vi "Main_HSI.vi"() -> ()   [LabVIEW 2018]
uses:
  <vilib>/vision/Image Controls.llb/IMAQ Image.ctl
  Hyperspectral_Analysis_v2018 - Copie/HSI.llb/Commande 1.ctl
panel:
  out "SPECTRUM ON ROI":cluster{"WAVELENGTH":dbl[], "SPECTRUM":dbl[]}[](graph)
  out "IMAGE U8":u8[][][](array[numeric])
  in  "BAND TO VISUALIZE 3":i32=45 caption="BAND TO VISUALIZE"
  in  "BAND TO VISUALIZE 2":i32=45 caption="BAND TO VISUALIZE"
  in  "GREEN BAND 3":i32=45 caption="GREEN BAND"
  in  "BLUE BAND 3":i32=45 caption="BLUE BAND"
  in  "RED BAND 3":i32=45 caption="RED BAND"
  in  "GREEN BAND 2":i32=45 caption="GREEN BAND"
  in  "BLUE BAND 2":i32=45 caption="BLUE BAND"
  in  "RED BAND 2":i32=45 caption="RED BAND"
  out "path 2":path
  out "path":path
  out "VISU RGB IMAGE":T1
  in  "GREEN BAND":i32=45
  in  "BLUE BAND":i32=45
  in  "RED BAND":i32=45
  out "DISPLAY RGB IMAGE":T1(plugin-control)
  in  "START SPECTRA CALCULATION":bool
  in  "BACK TO MAIN 3":bool
  in  "BACK TO MAIN 2":bool
  in  "IMAGES FOLDER":path
  out "SPECTRA OF CLUSTER CENTERS":cluster{"WAVELENGTH":dbl[], "SPECTRUM":dbl[]}[](graph)
  in  "XSTART":i16=1
  in  "# Clusters":i16=4
  in  "YEND":i16=300
  in  "XEND":i16=300
  in  "YSTART":i16=1
  in  "# Iterations":i16=100
  out "ANALYSIS IN PROGRESS":u16(slide) max=100 step=10 scale=0.0..100.0 scale format="%.1f"
  out "CLUSTER":T1(plugin-control)
  in  "CALCULATE CLUSTER":bool
  out "ROI":T2
  in  "IMAGE PATH":path
  out "CURRENT PICTURE ANALYZED":string
  in  "NEXT IMAGE":bool
  out "WAVELENGTH":sgl[](array[numeric])=[470.0, 472.8859, 475.7718, 478.6577, 481.5436, 484.4295, 487.3154, 490.2013, 493.0872, 495.9732, 498.8591, 501.745, 504.6309, 507.5168, 510.4027, 513.2886, 516.1745, 519.0604, 521.9463, 524.8322, 527.7181, 530.604, 533.4899, 536.3758, 539.2617, 542.1477, 545.0336, 547.9195, 550.8054, 553.6913, 556.5772, 559.4631, 562.349, 565.2349, 568.1208, 571.0067, 573.8926, 576.7785, 579.6644, 582.5503, 585.4362, 588.3221, 591.2081, 594.094, 596.9799, 599.8658, 602.7517, 605.6376, 608.5235, 611.4094, 614.2953, 617.1812, 620.0671, 622.953, 625.8389, 628.7248, 631.6107, 634.4966, 637.3826, 640.2685, 643.1544, 646.0403, 648.9262, 651.8121, 654.698, 657.5839, 660.4698, 663.3557, 666.2416, 669.1275, 672.0134, 674.8993, 677.7852, 680.6711, 683.557, 686.443, 689.3289, 692.2148, 695.1007, 697.9866, 700.8725, 703.7584, 706.6443, 709.5302, 712.4161, 715.302, 718.1879, 721.0738, 723.9597, 726.8456, 729.7315, 732.6174, 735.5034, 738.3893, 741.2752, 744.1611, 747.047, 749.9329, 752.8188, 755.7047, 758.5906, 761.4765, 764.3624, 767.2483, 770.1342, 773.0201, 775.906, 778.7919, 781.6779, 784.5638, 787.4497, 790.3356, 793.2215, 796.1074, 798.9933, 801.8792, 804.7651, 807.651, 810.5369, 813.4228, 816.3087, 819.1946, 822.0805, 824.9664, 827.8523, 830.7383, 833.6242, 836.5101, 839.396, 842.2819, 845.1678, 848.0537, 850.9396, 853.8255, 856.7114, 859.5973, 862.4832, 865.3691, 868.255, 871.1409, 874.0268, 876.9128, 879.7987, 882.6846, 885.5705, 888.4564, 891.3423, 894.2282, 897.1141, 900.0]
  out "CUBE":sgl[][][](array[numeric])
  in  "BACK TO MAIN":bool
  out "VISU 1 LAYER U8":T1
  in  "BAND TO VISUALIZE":i32=45
  in  "WAVELENGTH NUMBER":i32=150
  in  "IMAGES FOLDER PATH":path
  in  "START CLUSTERIZATION":bool
  out "DISPLAY 1 BAND":T1(plugin-control)
  in  "QUIT":bool=TRUE
  in  "ROI AUTO":bool=TRUE
  in  "DEMO":bool=TRUE
  in  "AVERAGE SPECTRUM":bool=TRUE
  in  "CLUSTERIZATION":bool
  # "Hyperspectral Analysis v1.0"
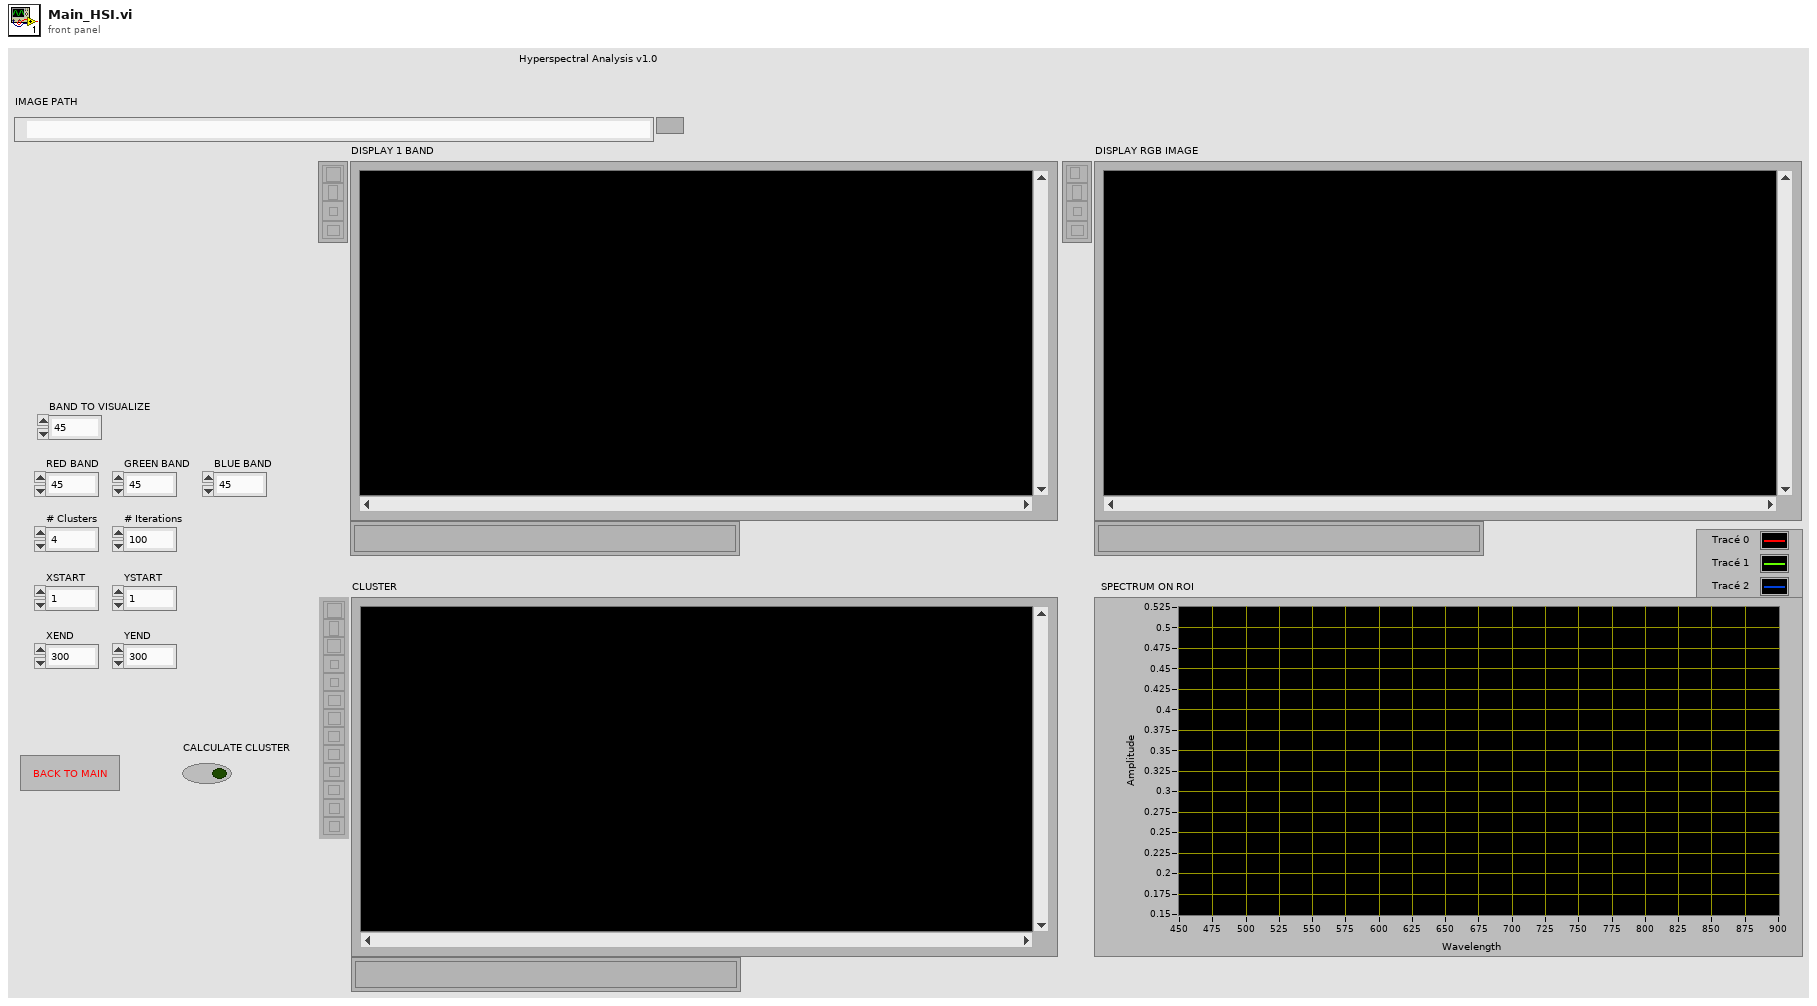
[diagram p1: front panel]
types:
  T1 = typedef "IMAQ Image.ctl" = refnum<image>
  T2 = cluster{"Global Rectangle":i32[], "Contours":cluster{"Contour Type":u32, "ROI Type":u32, "Points":i32[]}[]}
  T3 = enum8{"Enabled", "Disabled", "Disabled and Grayed Out"}
  T4 = typedef "Commande 1.ctl" = cluster{"Tableau":dbl[], "Tableau 2":dbl[]}[]
  T5 = typedef "Image Type" = u32
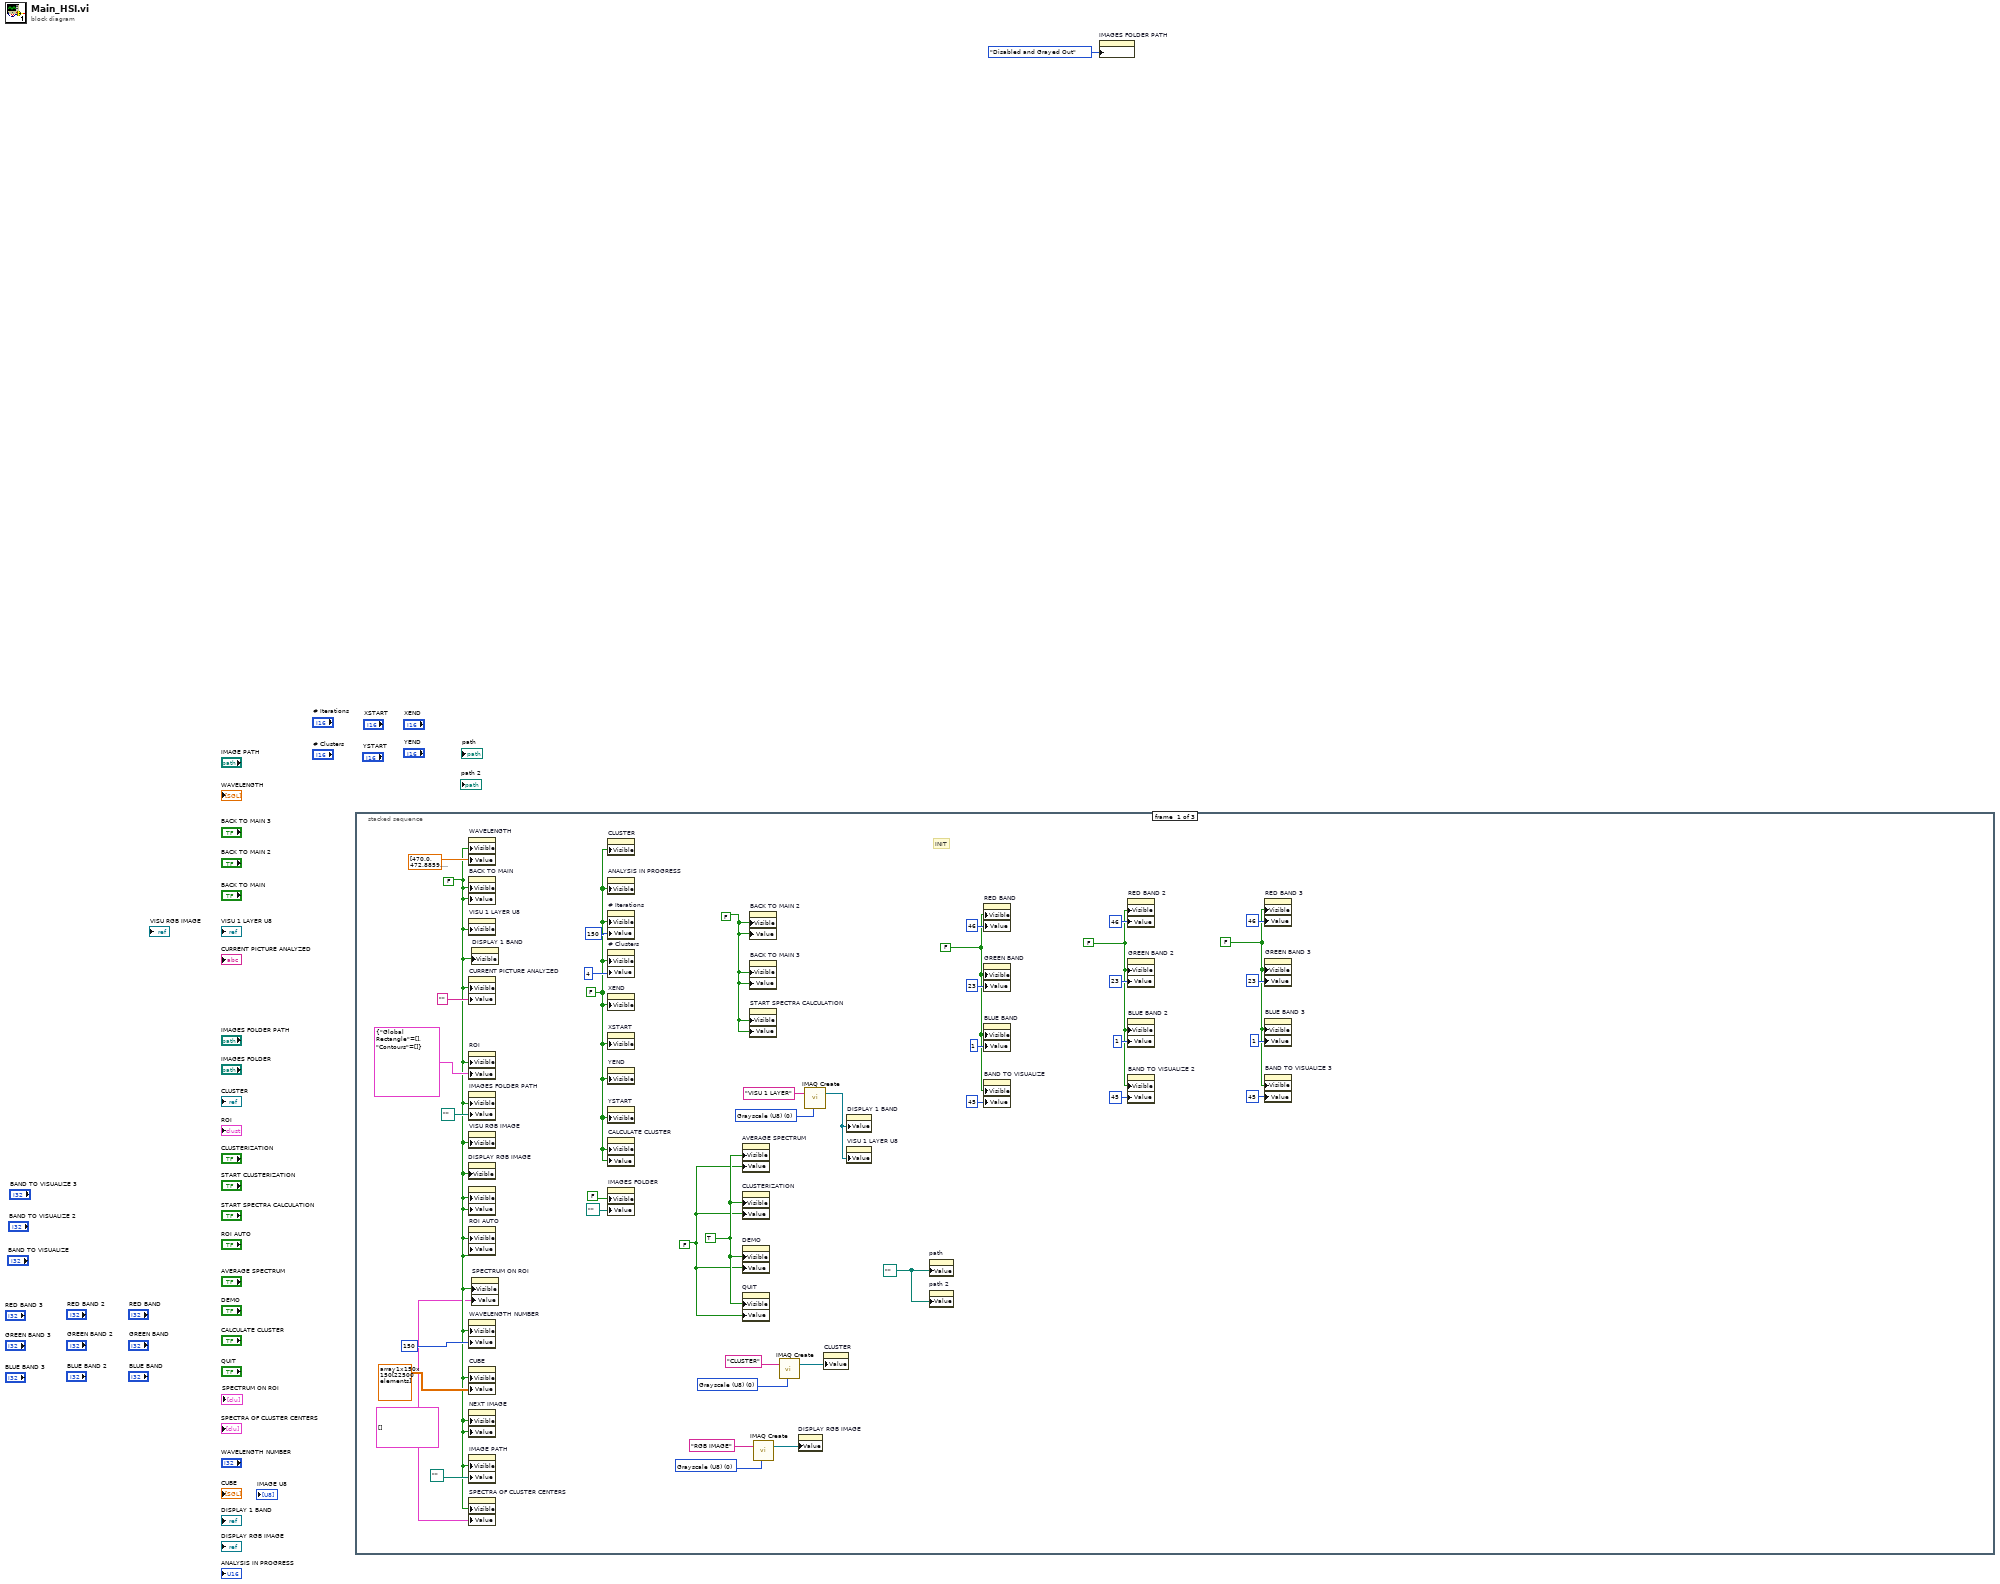
[diagram p0: block diagram]
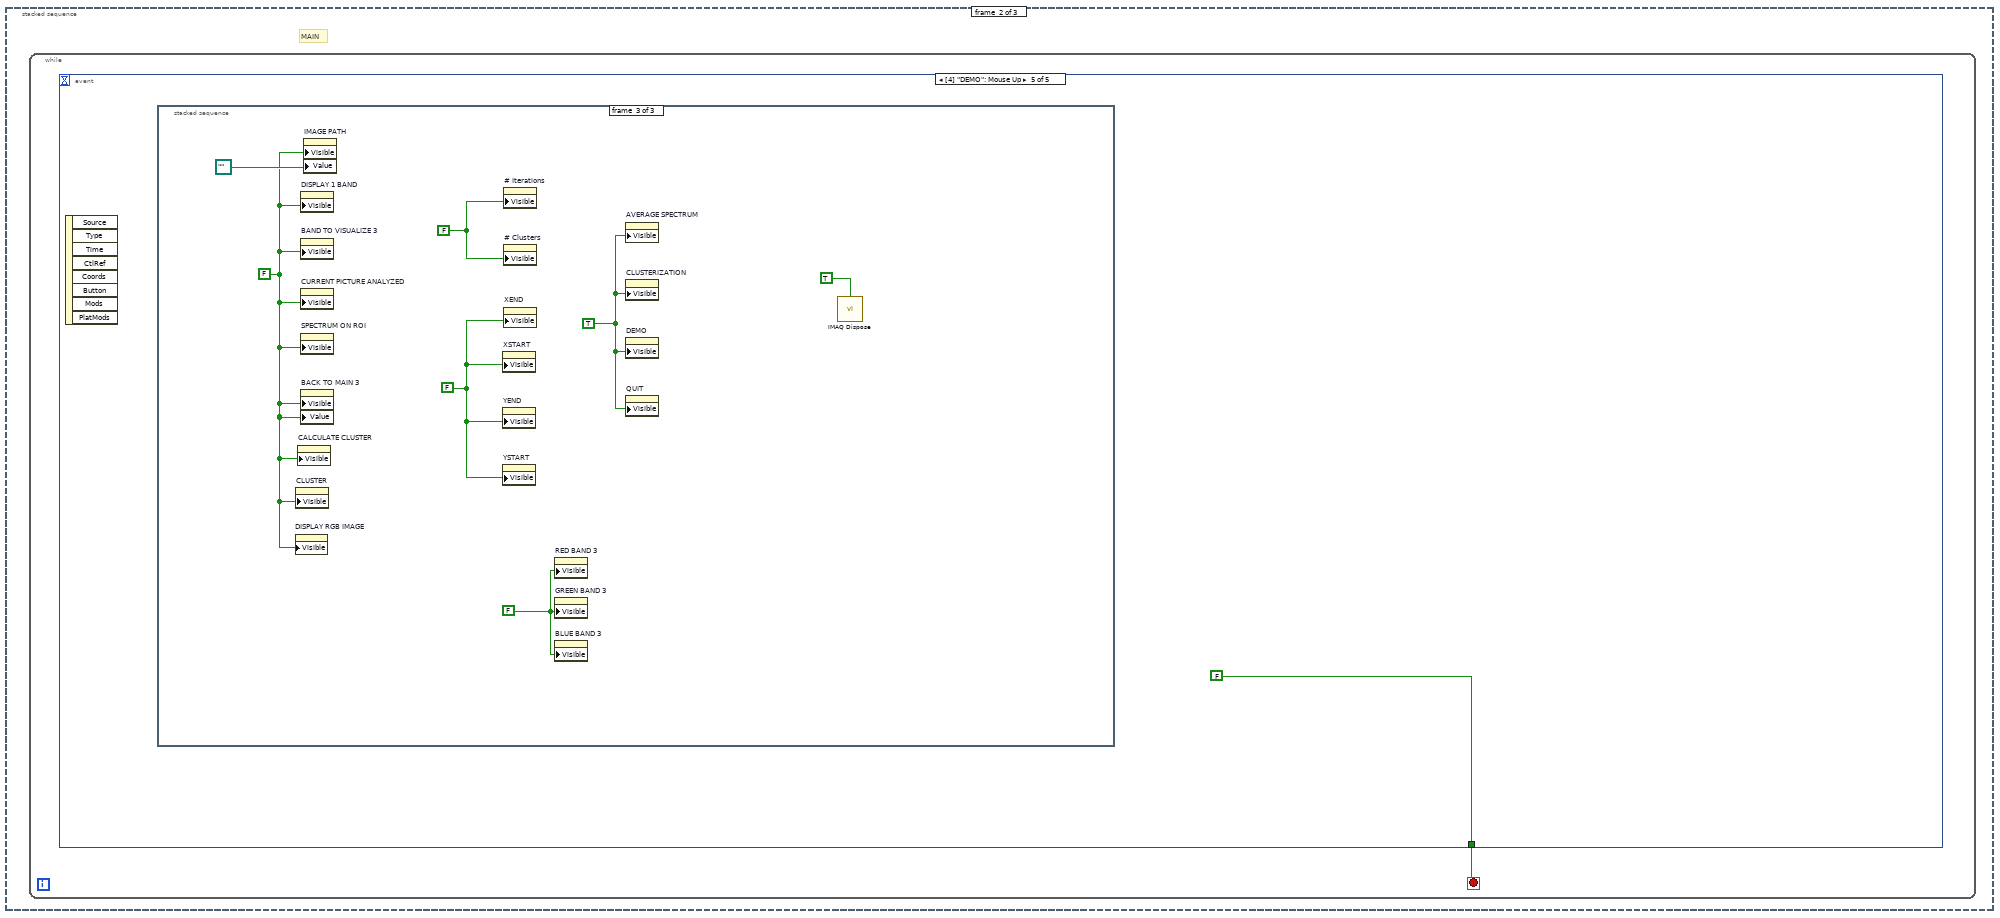
[diagram p2: hidden frame]
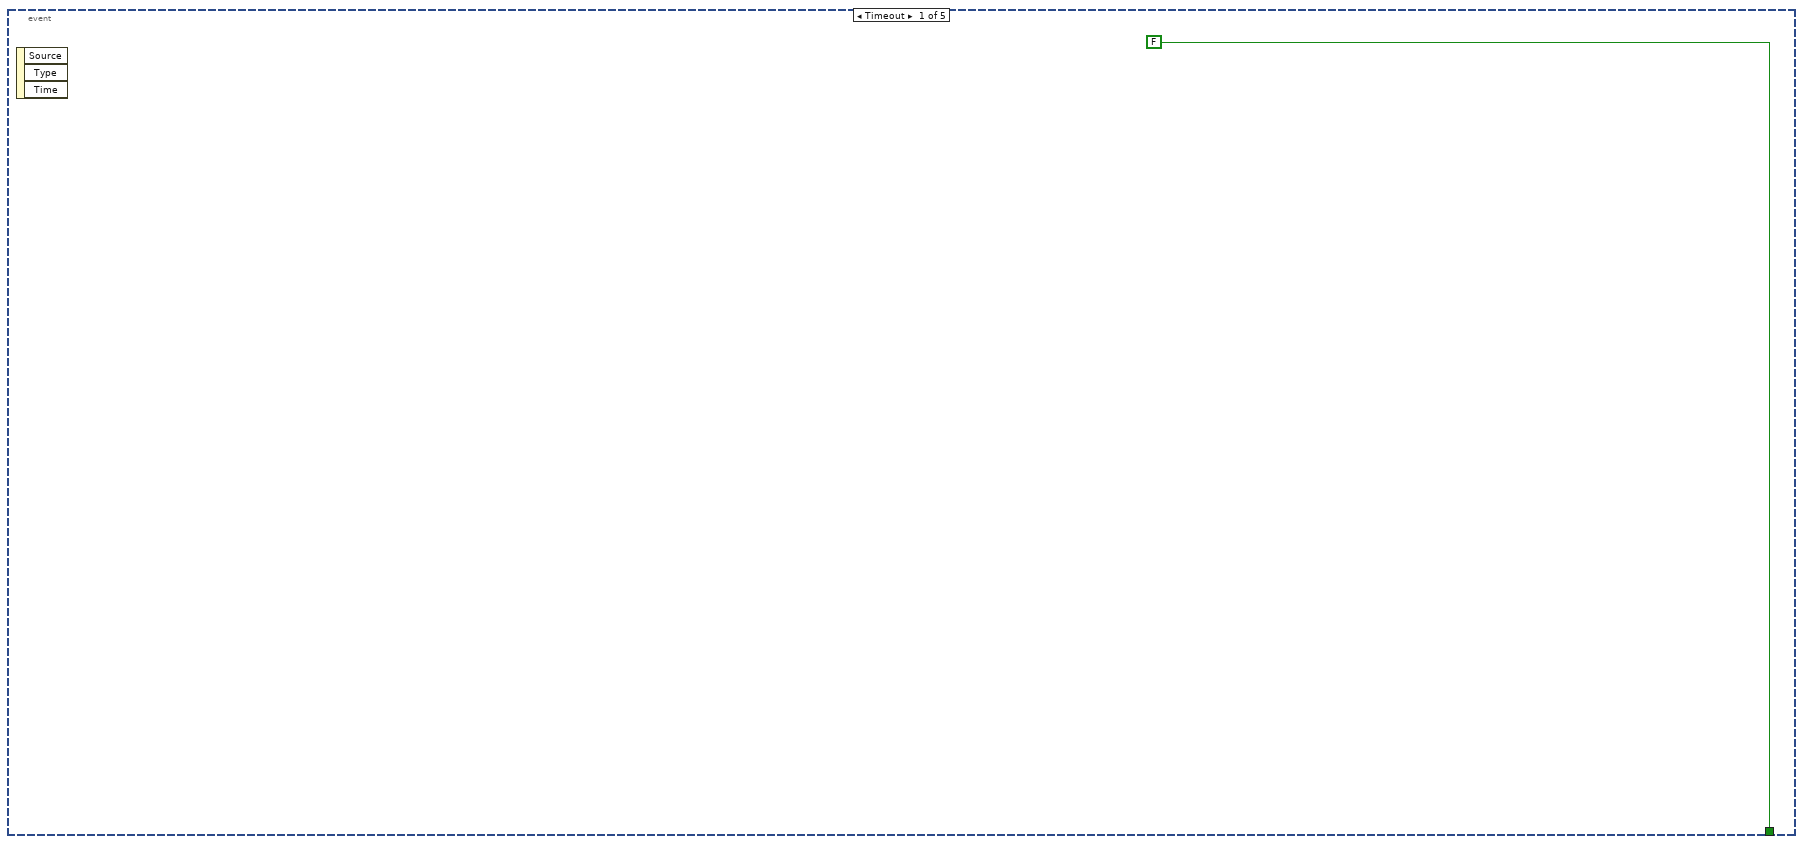
[diagram p3: hidden frame]
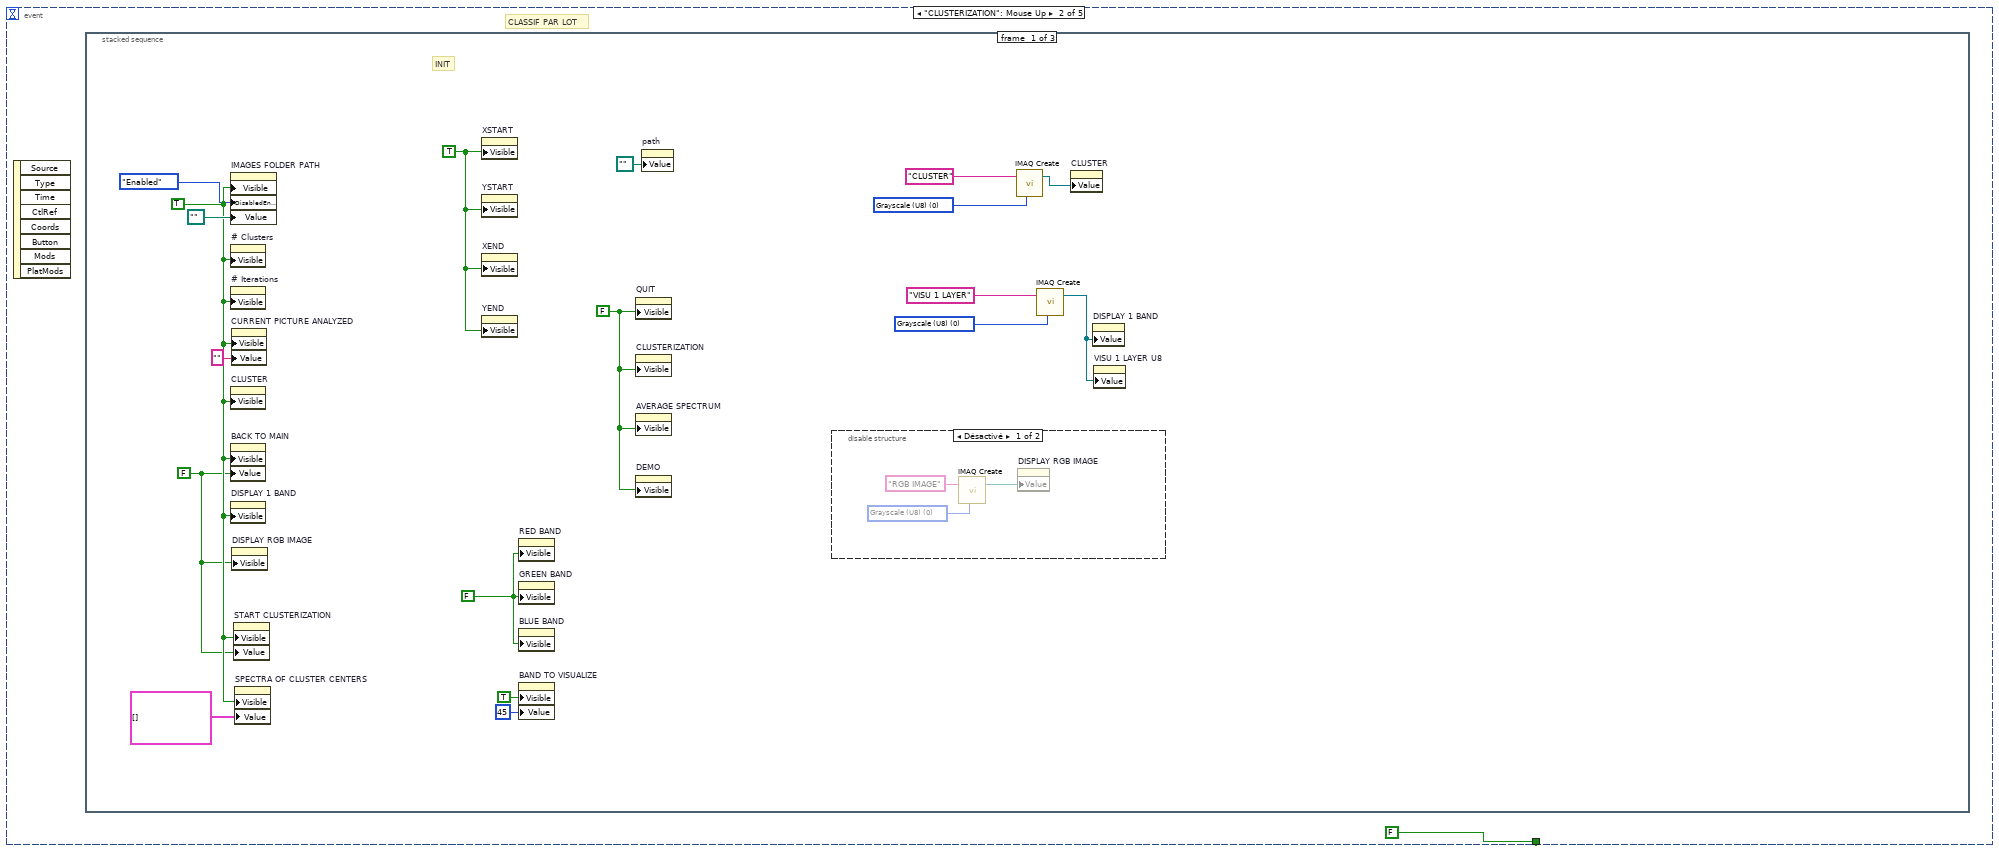
[diagram p4: hidden frame]
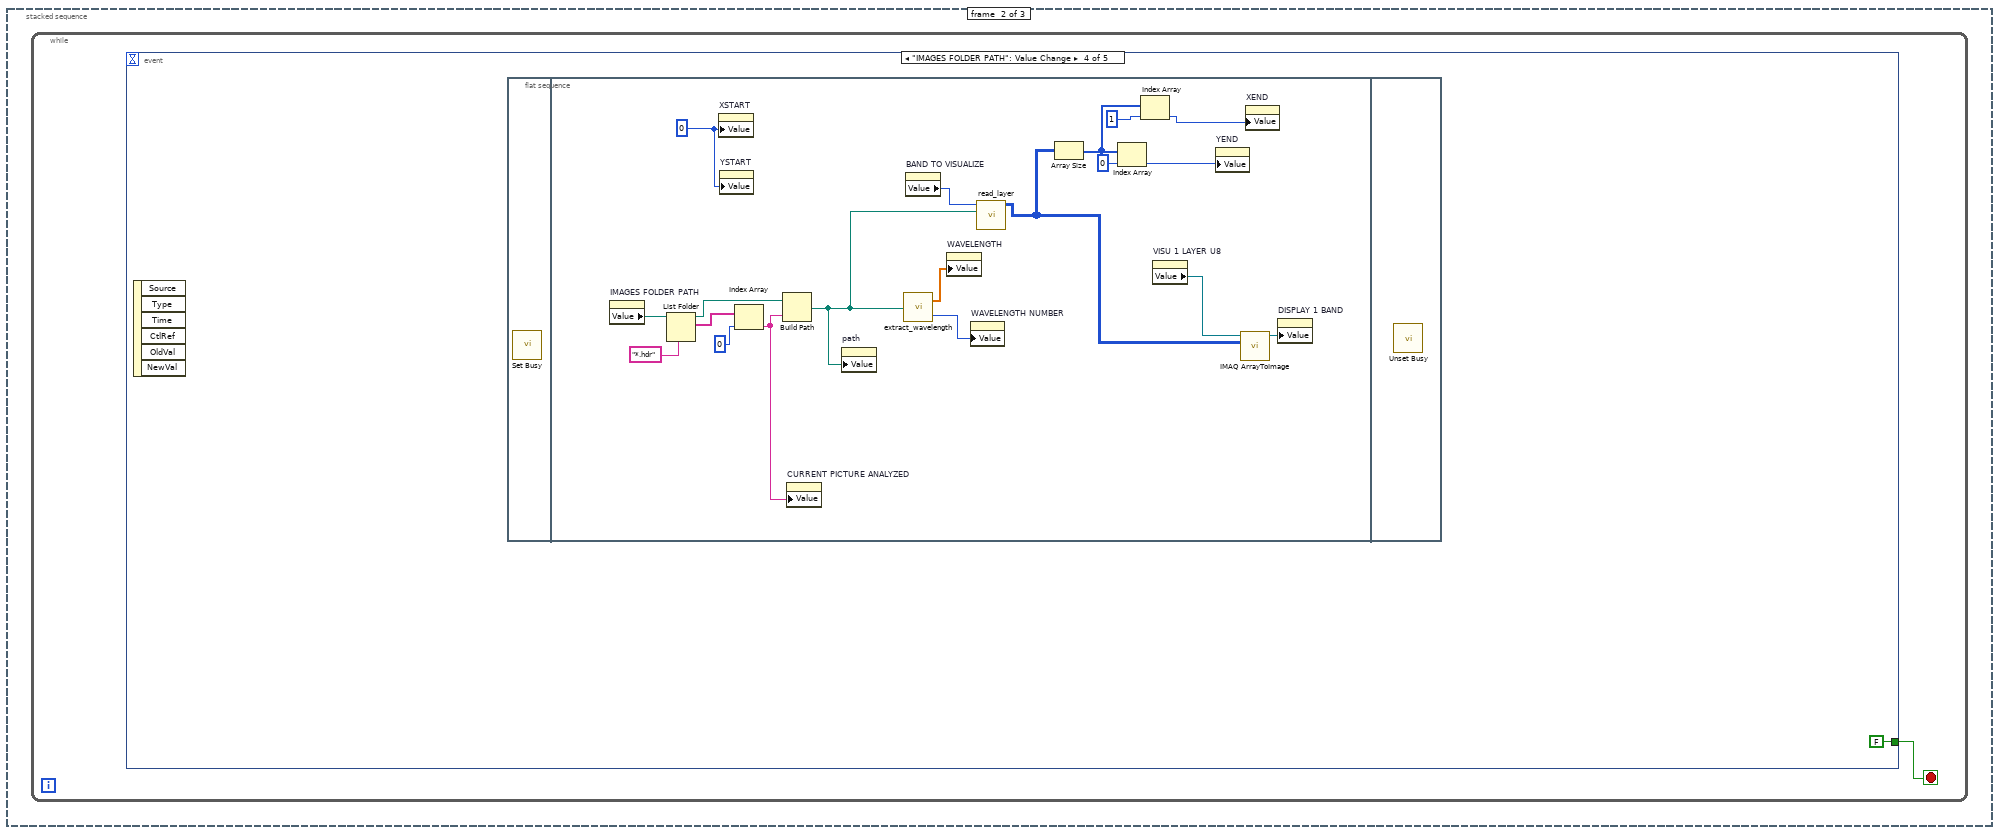
[diagram p6: hidden frame]
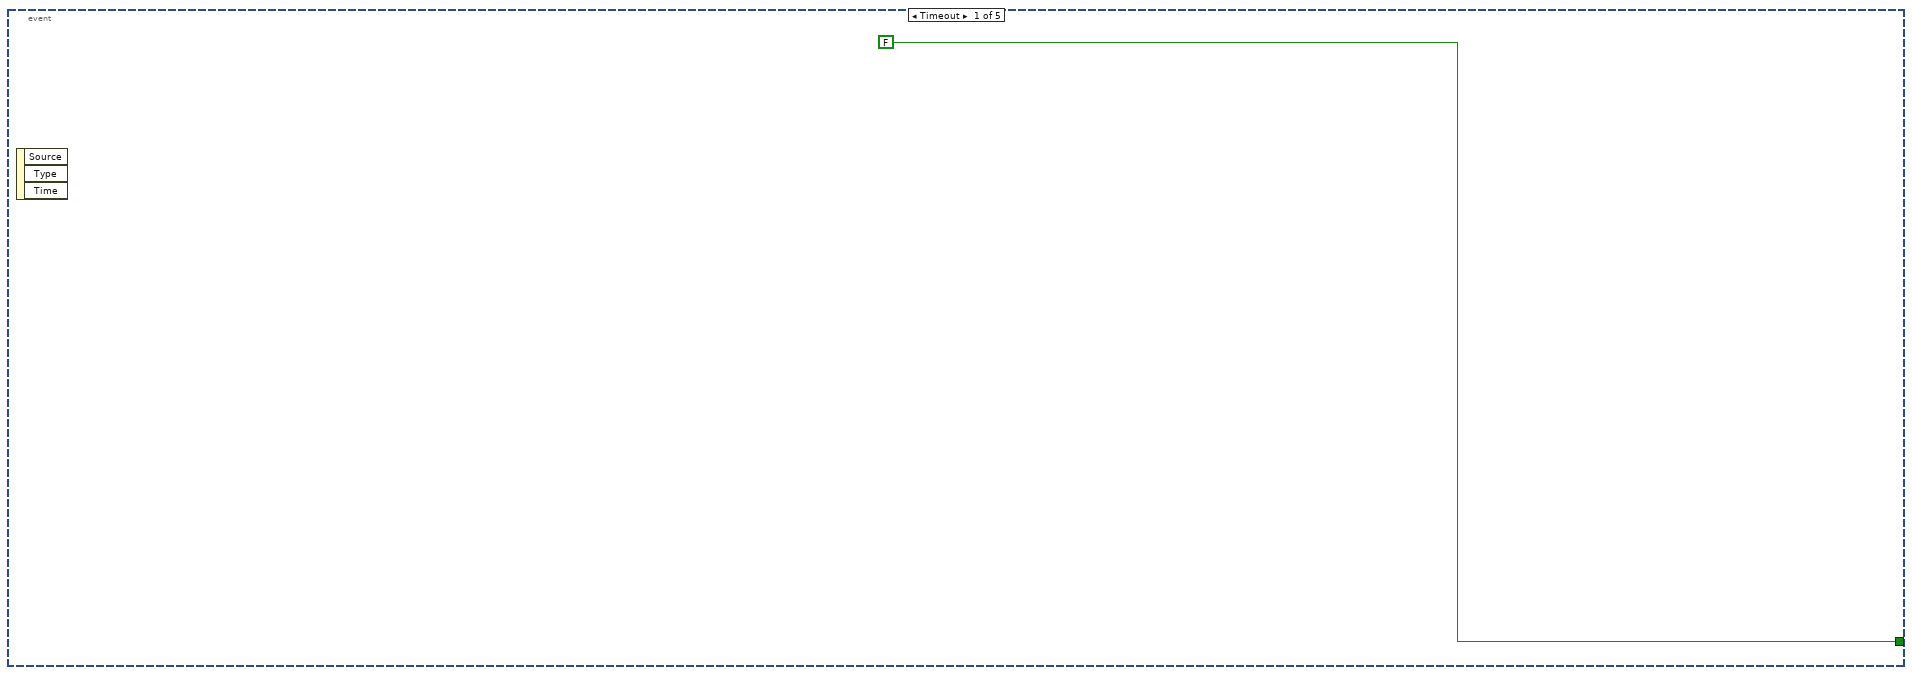
[diagram p7: hidden frame]
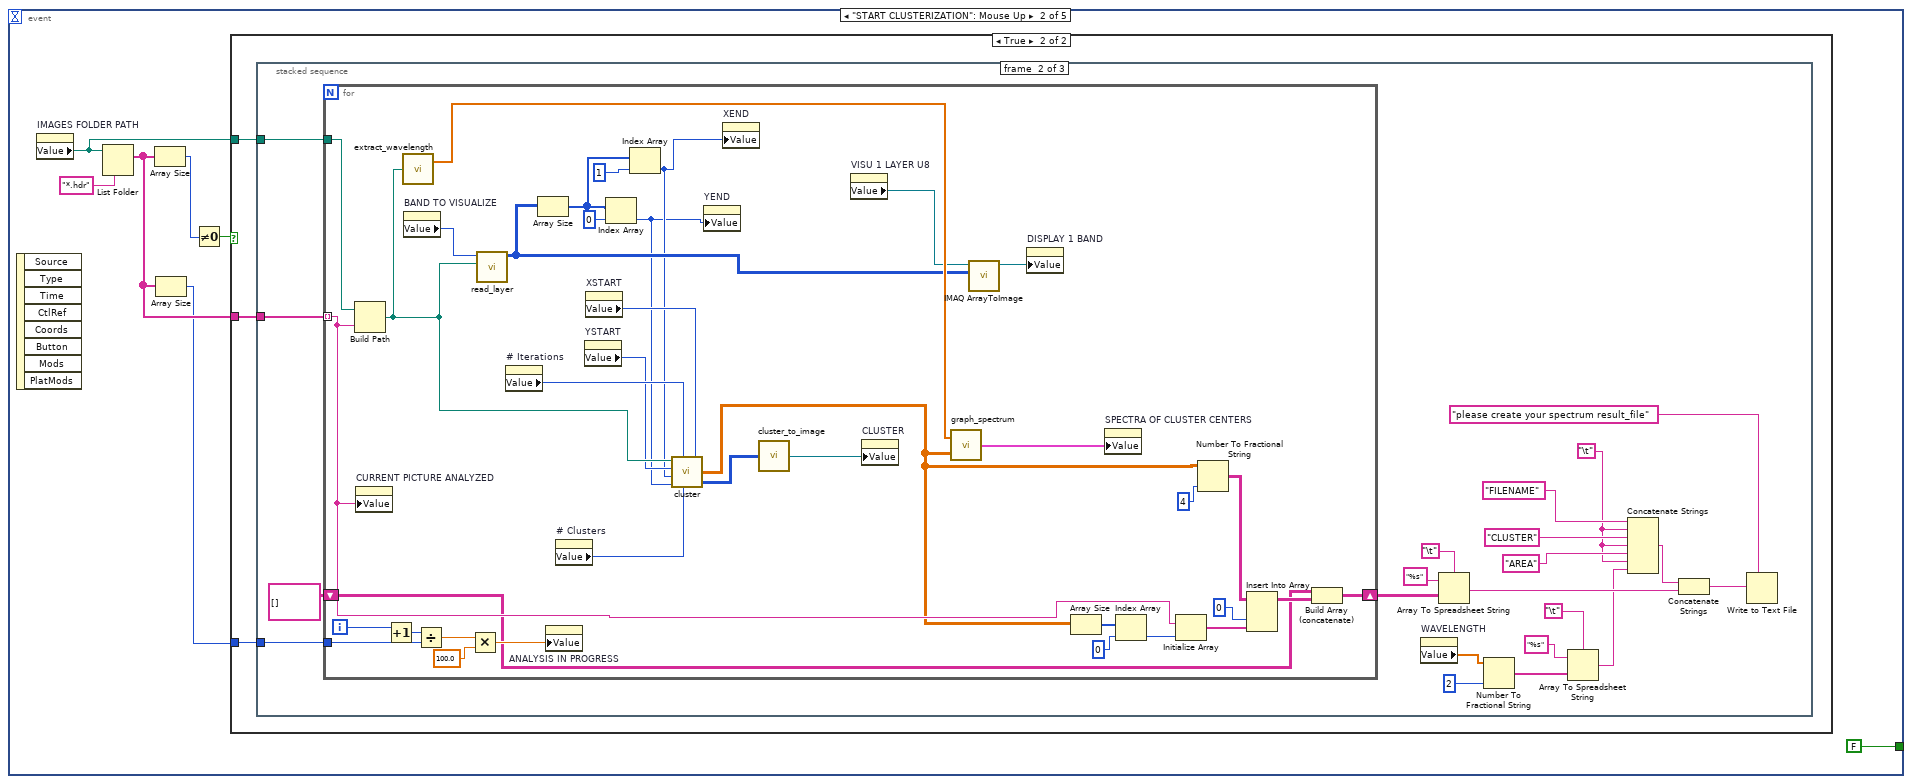
[diagram p8: hidden frame]
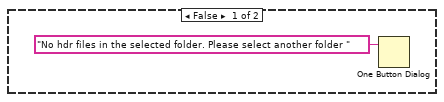
[diagram p9: hidden frame]
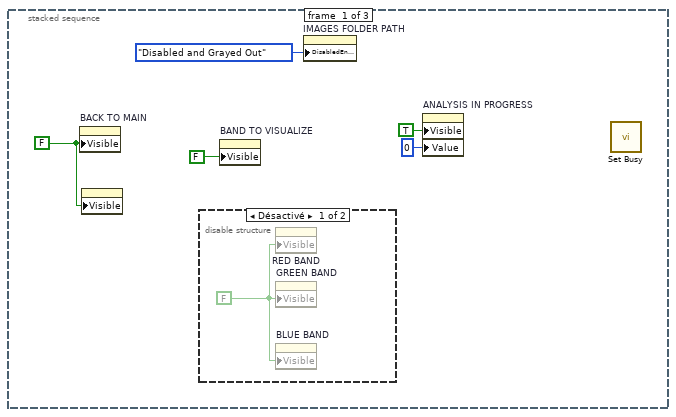
[diagram p10: hidden frame]
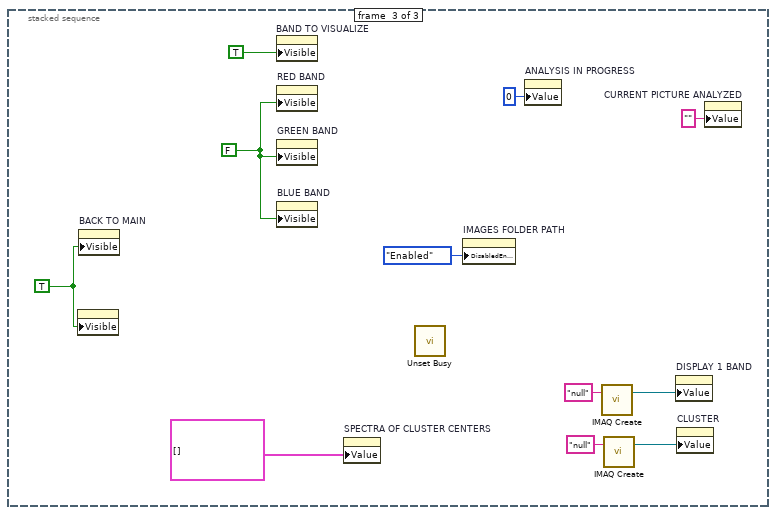
[diagram p12: hidden frame]
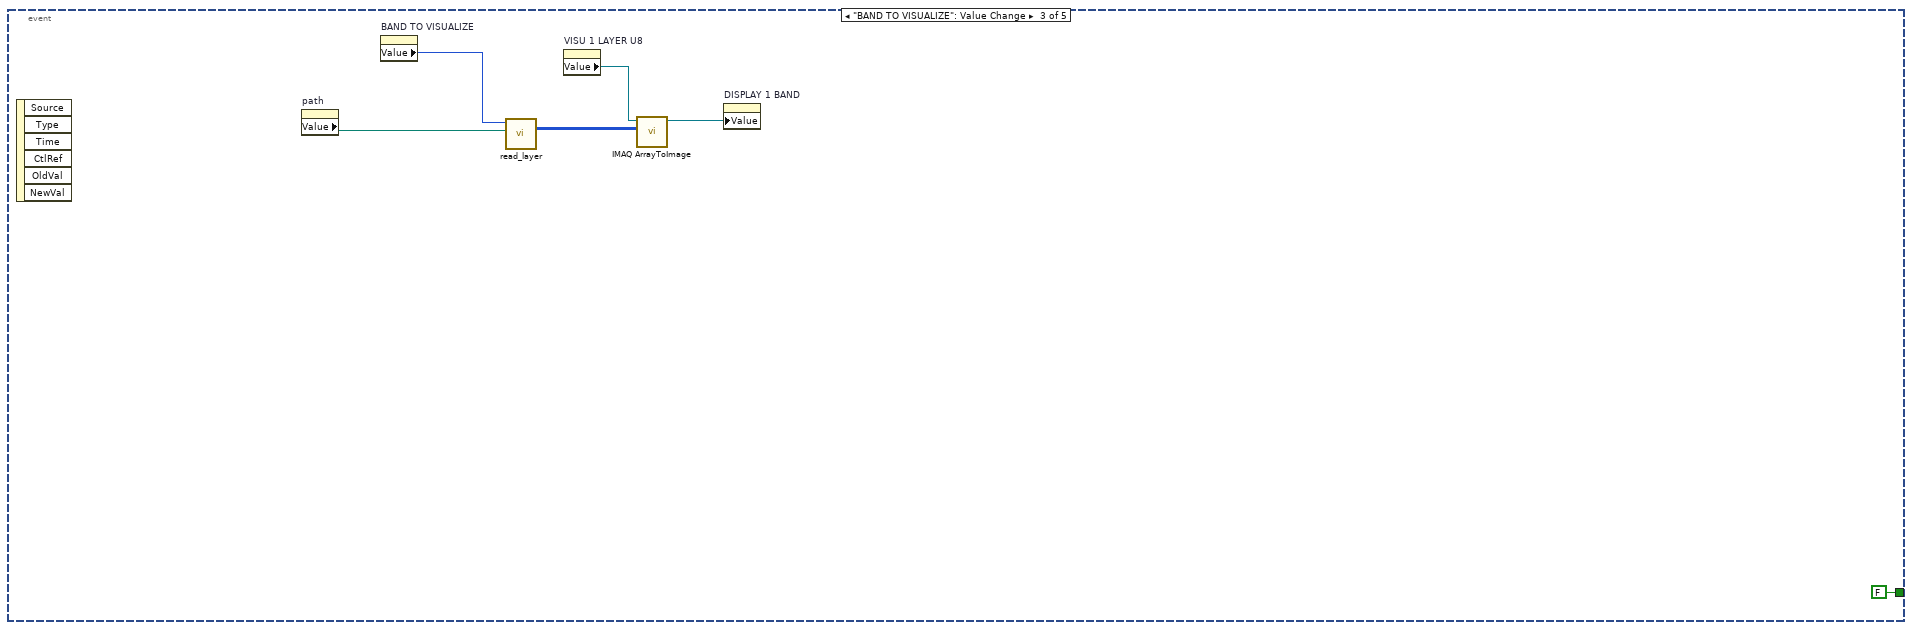
[diagram p13: hidden frame]
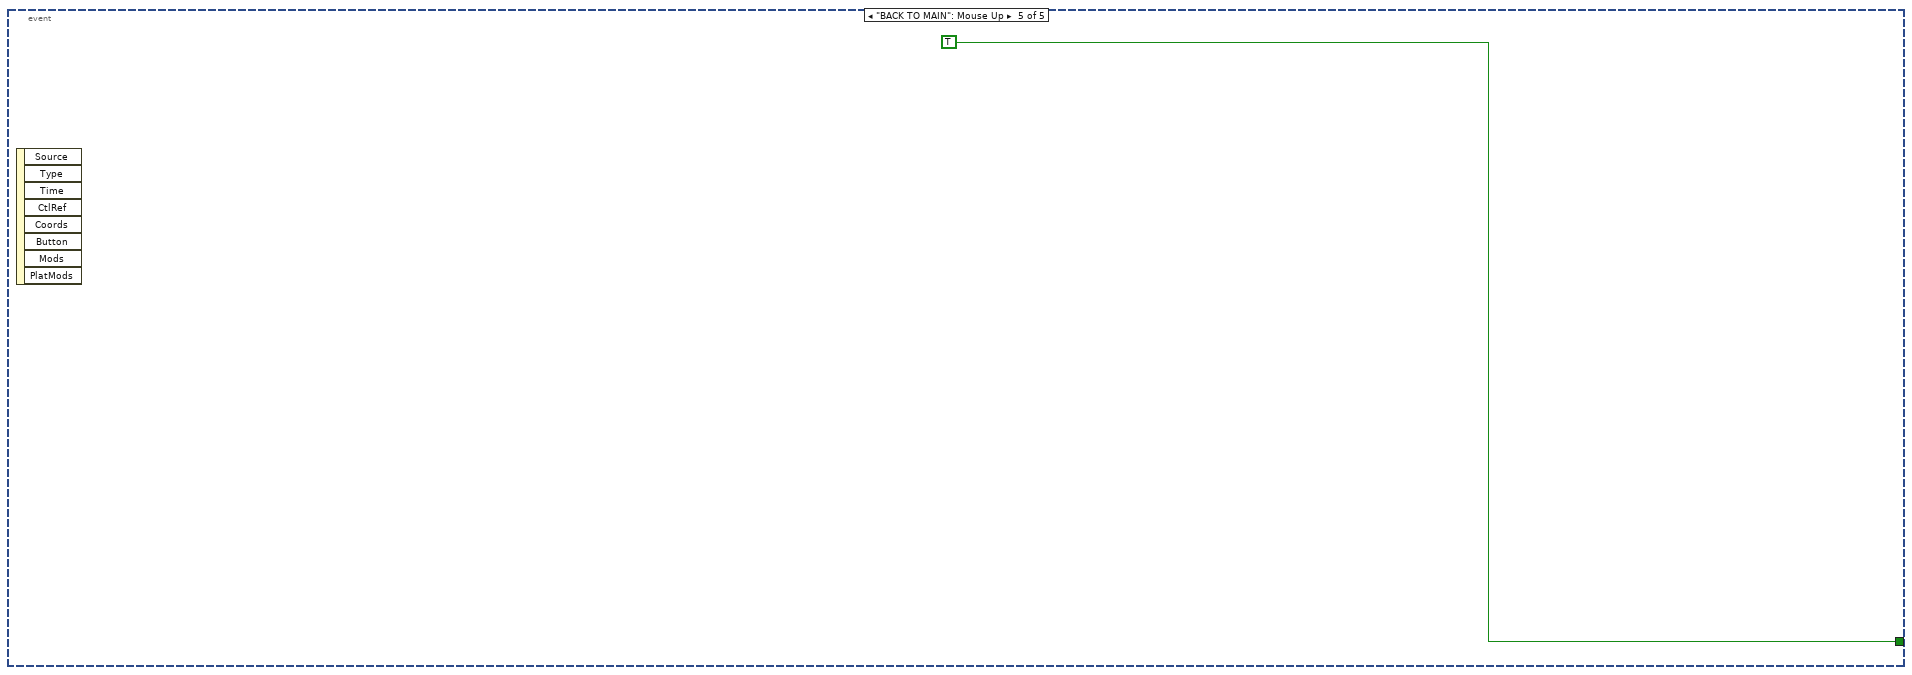
[diagram p14: hidden frame]
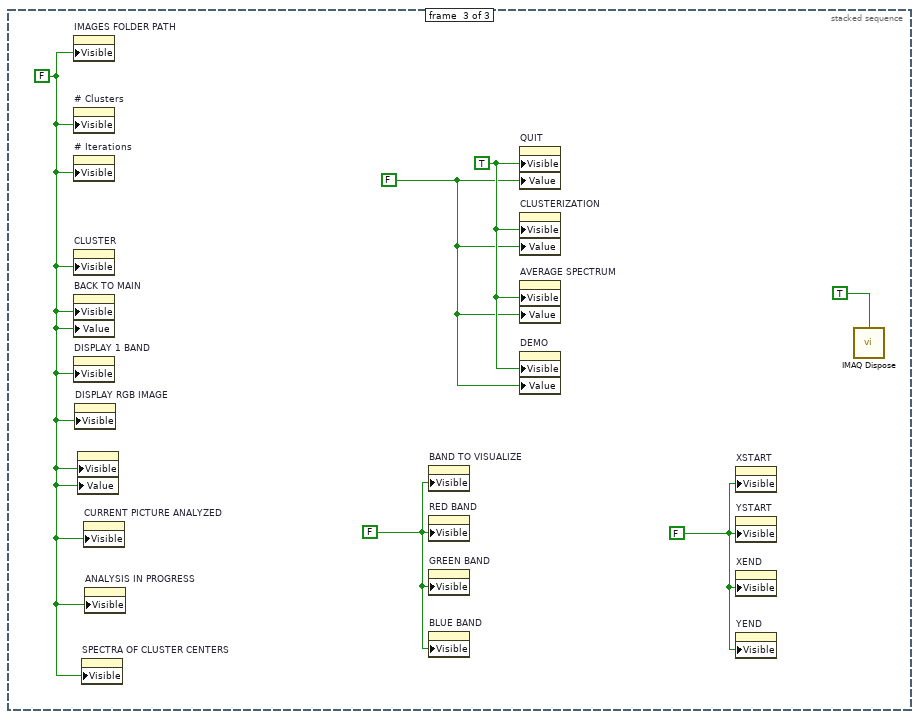
[diagram p15: hidden frame]
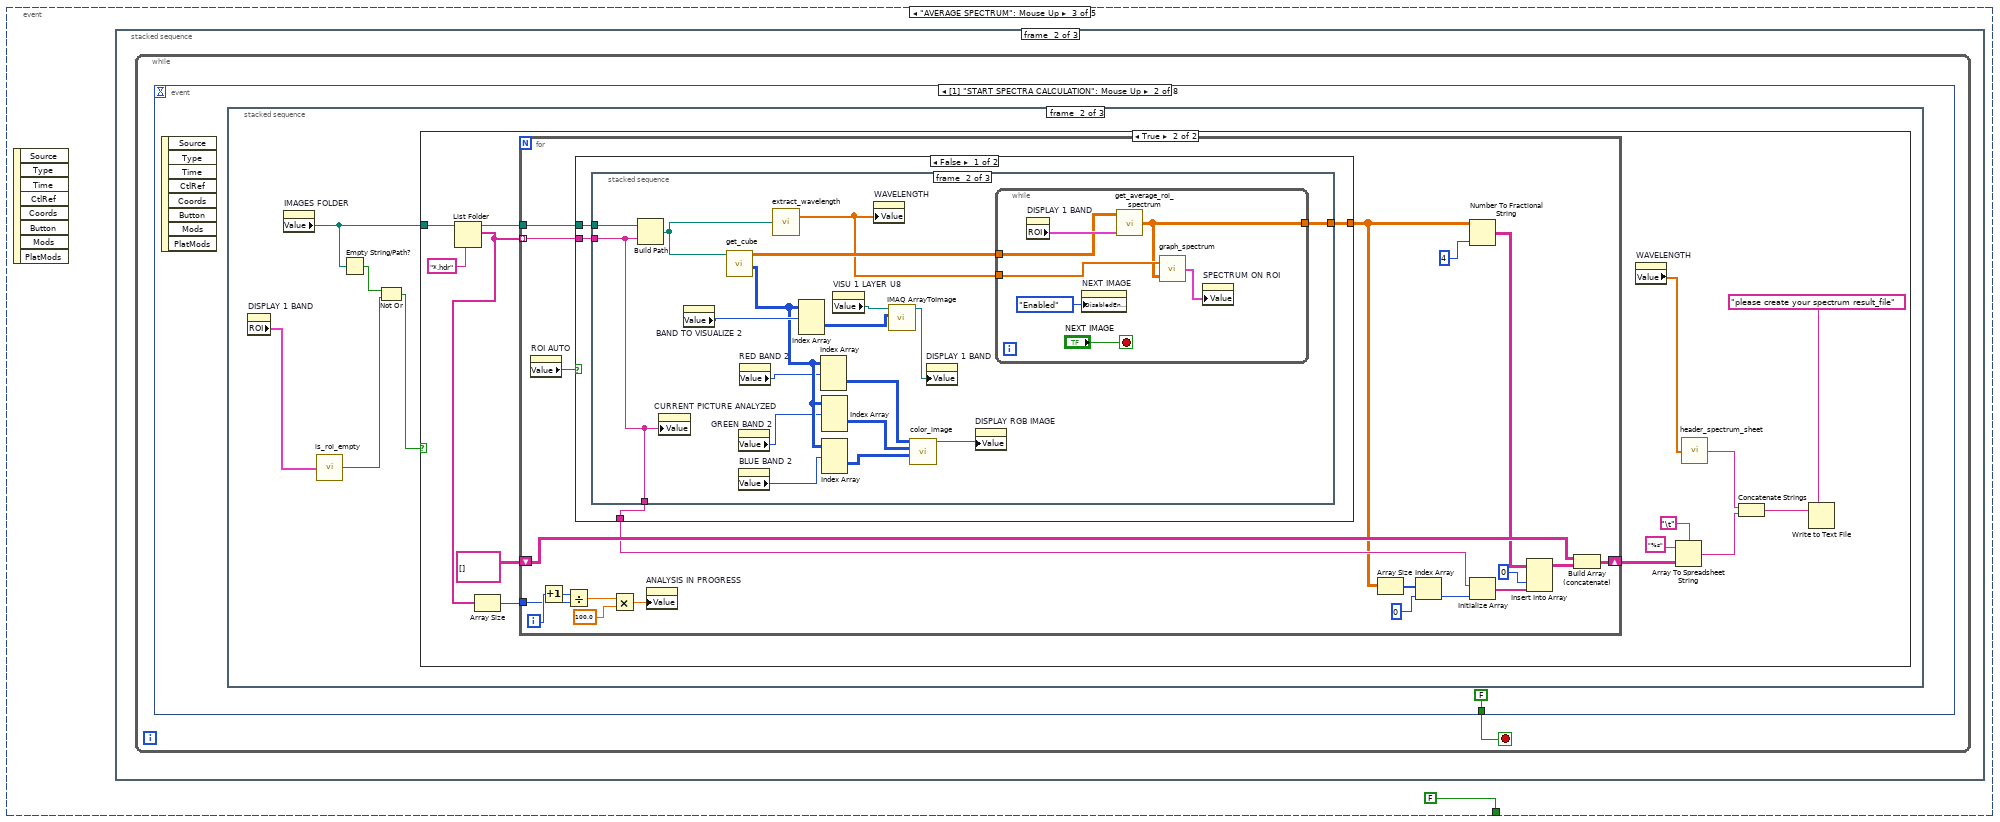
[diagram p16: hidden frame]
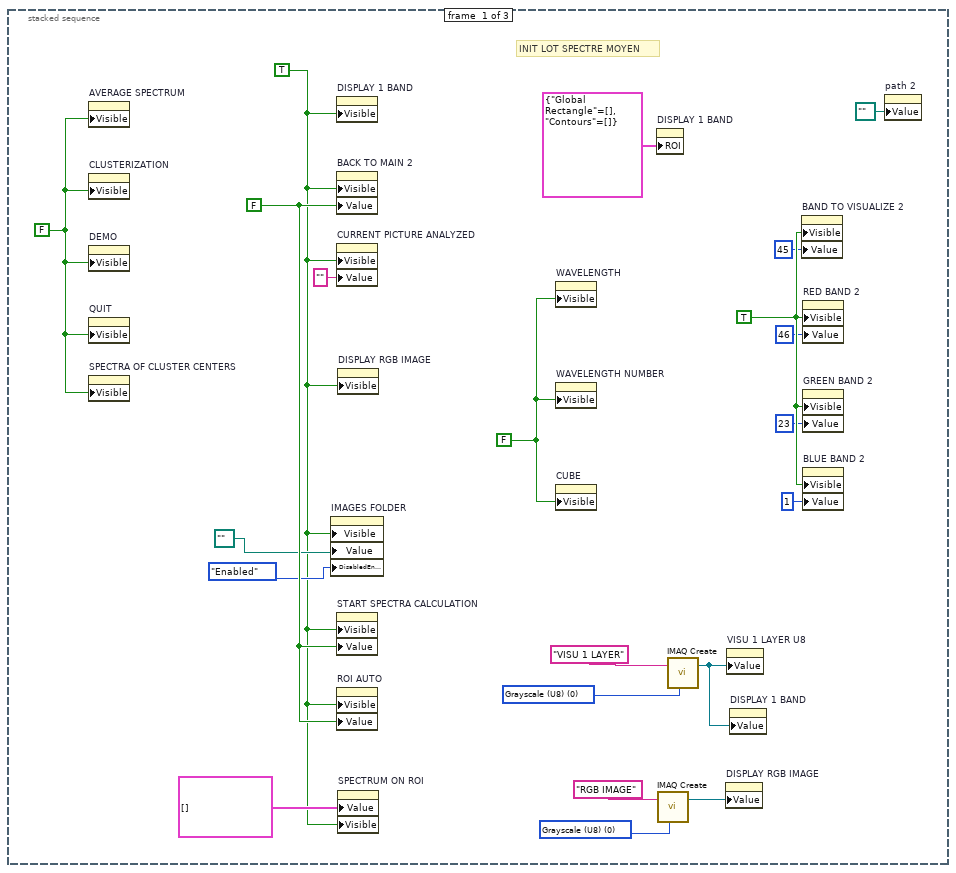
[diagram p17: hidden frame]
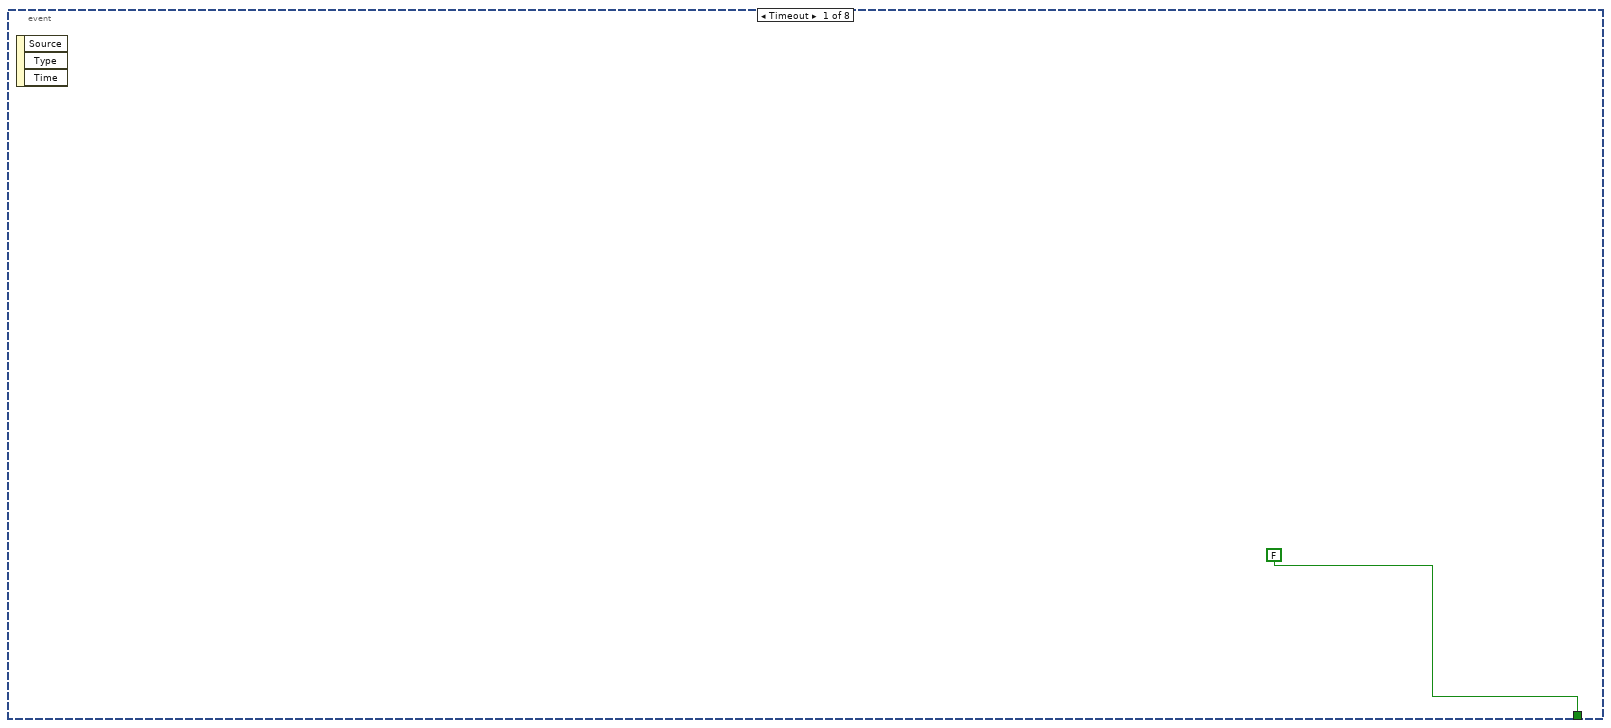
[diagram p18: hidden frame]
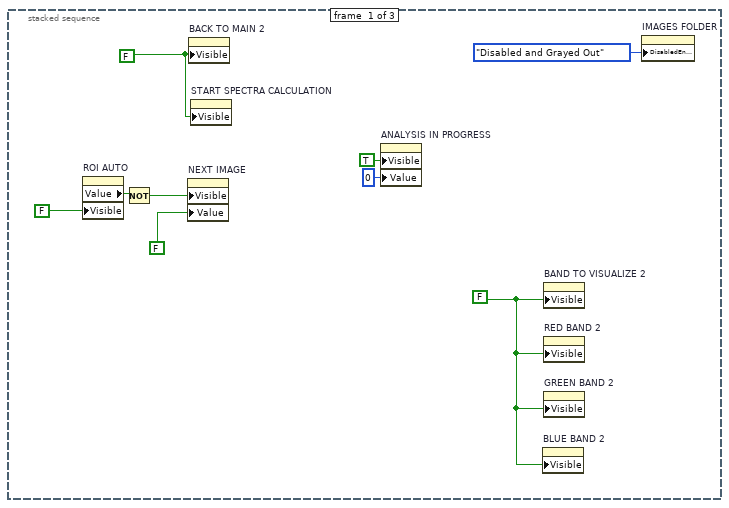
[diagram p19: hidden frame]
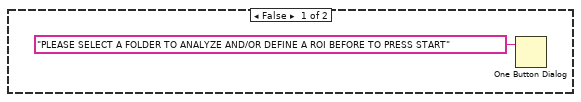
[diagram p20: hidden frame]
diagram:
  n1 = stacked-sequence {
    frame #0 {
      w5 = FALSE
      w10 = FALSE
      w14 = path "" ("path")
      w16 = FALSE
      w21 = T5 0 items=["Grayscale (U8)", "Grayscale (I16)", "Grayscale (SGL)", "Complex (CSG)", "RGB (U32)", "HSL (U32)", "RGB (U64)", "Grayscale (U16)"] ("Image Type")
      w24 = T5 0 items=["Grayscale (U8)", "Grayscale (I16)", "Grayscale (SGL)", "Complex (CSG)", "RGB (U32)", "HSL (U32)", "RGB (U64)", "Grayscale (U16)"] ("Image Type")
      w27 = TRUE
      w29 = FALSE
      w32 = T5 0 items=["Grayscale (U8)", "Grayscale (I16)", "Grayscale (SGL)", "Complex (CSG)", "RGB (U32)", "HSL (U32)", "RGB (U64)", "Grayscale (U16)"] ("Image Type")
      w2 = T4 [] ("SPECTRUM ON ROI")
      w26 = FALSE ("AVERAGE SPECTRUM")
      w28 = FALSE
      w3 = FALSE
      # "INIT"
      n2 = property on="DISPLAY RGB IMAGE" class="ImageControl"("Visible"=w3) -> ()  [unwired: 2 in, 2 out]
      n3 = property on="WAVELENGTH" class="Arr (strict)"("Visible"=w3, "Value"=dbl[] [470.0, 472.8859, 475.7718, 478.6577, 481.5436, 484.4295, 487.3154, 490.2013, 493.0872, 495.9732, 498.8591, 501.745, 504.6309, 507.5168, 510.4027, 513.2886, 516.1745, 519.0604, 521.9463, 524.8322, 527.7181, 530.604, 533.4899, 536.3758, 539.2617, 542.1477, 545.0336, 547.9195, 550.8054, 553.6913, 556.5772, 559.4631, 562.349, 565.2349, 568.1208, 571.0067, 573.8926, 576.7785, 579.6644, 582.5503, 585.4362, 588.3221, 591.2081, 594.094, 596.9799, 599.8658, 602.7517, 605.6376, 608.5235, 611.4094, 614.2953, 617.1812, 620.0671, 622.953, 625.8389, 628.7248, 631.6107, 634.4966, 637.3826, 640.2685, 643.1544, 646.0403, 648.9262, 651.8121, 654.698, 657.5839, 660.4698, 663.3557, 666.2416, 669.1275, 672.0134, 674.8993, 677.7852, 680.6711, 683.557, 686.443, 689.3289, 692.2148, 695.1007, 697.9866, 700.8725, 703.7584, 706.6443, 709.5302, 712.4161, 715.302, 718.1879, 721.0738, 723.9597, 726.8456, 729.7315, 732.6174, 735.5034, 738.3893, 741.2752, 744.1611, 747.047, 749.9329, 752.8188, 755.7047, 758.5906, 761.4765, 764.3624, 767.2483, 770.1342, 773.0201, 775.906, 778.7919, 781.6779, 784.5638, 787.4497, 790.3356, 793.2215, 796.1074, 798.9933, 801.8792, 804.7651, 807.651, 810.5369, 813.4228, 816.3087, 819.1946, 822.0805, 824.9664, 827.8523, 830.7383, 833.6242, 836.5101, 839.396, 842.2819, 845.1678, 848.0537, 850.9396, 853.8255, 856.7114, 859.5973, 862.4832, 865.3691, 868.255, 871.1409, 874.0268, 876.9128, 879.7987, 882.6846, 885.5705, 888.4564, 891.3423, 894.2282, 897.1141, 900.0] ("WAVELENGTH")) -> ()  [unwired: 2 in, 2 out]
      n4 = property on="BACK TO MAIN" class="Bool (strict)"("Visible"=w3, "Value"=w3) -> ()  [unwired: 2 in, 2 out]
      n5 = property on="VISU 1 LAYER U8" class="IMAQImage (strict)"("Visible"=w3) -> ()  [unwired: 2 in, 2 out]
      n6 = property on="CURRENT PICTURE ANALYZED" class="Str"("Visible"=w3, "Value"="" ("CURRENT PICTURE ANALYZED")) -> ()  [unwired: 2 in, 2 out]
      n7 = property on="ROI" class="Clust (strict)"("Visible"=w3, "Value"=T2 {"Global Rectangle"=[], "Contours"=[]} ("ROI")) -> ()  [unwired: 2 in, 2 out]
      n8 = property on="IMAGES FOLDER PATH" class="Path"("Visible"=w3, "Value"=path "" ("IMAGES FOLDER PATH")) -> ()  [unwired: 2 in, 2 out]
      n9 = property on="VISU RGB IMAGE" class="IMAQImage (strict)"("Visible"=w3) -> ()  [unwired: 2 in, 2 out]
      n10 = property on="START CLUSTERIZATION" class="Bool (strict)"("Visible"=w3, "Value"=w3) -> ()  [unwired: 2 in, 2 out]
      n11 = property on="ROI AUTO" class="Bool (strict)"("Visible"=w3, "Value"=w3) -> ()  [unwired: 2 in, 2 out]
      n12 = property on="WAVELENGTH NUMBER" class="DigNum (strict)"("Visible"=w3, "Value"=150 ("WAVELENGTH NUMBER")) -> ()  [unwired: 2 in, 2 out]
      n13 = property on="CUBE" class="Arr (strict)"("Visible"=w3, "Value"=sgl[][][] array1x150x150[22500 elements] ("CUBE IMAGE")) -> ()  [unwired: 2 in, 2 out]
      n14 = property on="NEXT IMAGE" class="Bool (strict)"("Visible"=w3, "Value"=w3) -> ()  [unwired: 2 in, 2 out]
      n15 = property on="IMAGE PATH" class="Path"("Visible"=w3, "Value"=path "" ("IMAGES FOLDER PATH")) -> ()  [unwired: 2 in, 2 out]
      n16 = property on="SPECTRA OF CLUSTER CENTERS" class="XYGraph (strict)"("Visible"=w3, "Value"=w2) -> ()  [unwired: 2 in, 2 out]
      n17 = property on="DISPLAY 1 BAND" class="ImageControl"("Visible"=w3) -> ()  [unwired: 2 in, 2 out]
      n18 = property on="SPECTRUM ON ROI" class="XYGraph (strict)"("Visible"=w3, "Value"=w2) -> ()  [unwired: 2 in, 2 out]
      n19 = property on="CLUSTER" class="ImageControl"("Visible"=w28) -> ()  [unwired: 2 in, 2 out]
      n20 = property on="ANALYSIS IN PROGRESS" class="Slide (strict)"("Visible"=w28) -> ()  [unwired: 2 in, 2 out]
      n21 = property on="# Iterations" class="DigNum (strict)"("Visible"=w28, "Value"=i16 150 ("Nb Iteration")) -> ()  [unwired: 2 in, 2 out]
      n22 = property on="# Clusters" class="DigNum (strict)"("Visible"=w28, "Value"=i16 4 ("Nb Cluster")) -> ()  [unwired: 2 in, 2 out]
      n23 = property on="XEND" class="DigNum (strict)"("Visible"=w28) -> ()  [unwired: 2 in, 2 out]
      n24 = property on="XSTART" class="DigNum (strict)"("Visible"=w28) -> ()  [unwired: 2 in, 2 out]
      n25 = property on="YEND" class="DigNum (strict)"("Visible"=w28) -> ()  [unwired: 2 in, 2 out]
      n26 = property on="YSTART" class="DigNum (strict)"("Visible"=w28) -> ()  [unwired: 2 in, 2 out]
      n27 = property on="CALCULATE CLUSTER" class="Bool (strict)"("Visible"=w28, "Value"=w28) -> ()  [unwired: 2 in, 2 out]
      n28 = property on="IMAGES FOLDER" class="Path"("Visible"=FALSE, "Value"=path "" ("IMAGES FOLDER PATH 2")) -> ()  [unwired: 2 in, 2 out]
      n29 = property on="AVERAGE SPECTRUM" class="Bool (strict)"("Visible"=w27, "Value"=w26) -> ()  [unwired: 2 in, 2 out]
      n30 = property on="CLUSTERIZATION" class="Bool (strict)"("Visible"=w27, "Value"=w26) -> ()  [unwired: 2 in, 2 out]
      n31 = property on="DEMO" class="Bool (strict)"("Visible"=w27, "Value"=w26) -> ()  [unwired: 2 in, 2 out]
      n32 = property on="QUIT" class="Bool (strict)"("Visible"=w27, "Value"=w26) -> ()  [unwired: 2 in, 2 out]
      n33 = property on="BACK TO MAIN 2" class="Bool (strict)"("Visible"=w29, "Value"=w29) -> ()  [unwired: 2 in, 2 out]
      n34 = property on="BACK TO MAIN 3" class="Bool (strict)"("Visible"=w29, "Value"=w29) -> ()  [unwired: 2 in, 2 out]
      n35 = property on="START SPECTRA CALCULATION" class="Bool (strict)"("Visible"=w29, "Value"=w29) -> ()  [unwired: 2 in, 2 out]
      n36 = call "IMAQ Create"("Image Name"="RGB IMAGE", "Image Type"=w21) -> ("New Image"=w20:T1)  [unwired: 3 in, 1 out]
      n37 = call "IMAQ Create"("Image Name"="CLUSTER", "Image Type"=w24) -> ("New Image"=w23:T1)  [unwired: 3 in, 1 out]
      n38 = property on="DISPLAY RGB IMAGE" class="ImageControl"("Value"=w20) -> ()  [unwired: 2 in, 2 out]
      n39 = call "IMAQ Create"("Image Name"="VISU 1 LAYER", "Image Type"=w32) -> ("New Image"=w34:T1)  [unwired: 3 in, 1 out]
      n40 = property on="CLUSTER" class="ImageControl"("Value"=w23) -> ()  [unwired: 2 in, 2 out]
      n41 = property on="DISPLAY 1 BAND" class="ImageControl"("Value"=w34) -> ()  [unwired: 2 in, 2 out]
      n42 = property on="VISU 1 LAYER U8" class="IMAQImage (strict)"("Value"=w34) -> ()  [unwired: 2 in, 2 out]
      n43 = property on="path" class="Path"("Value"=w14) -> ()  [unwired: 2 in, 2 out]
      n44 = property on="path 2" class="Path"("Value"=w14) -> ()  [unwired: 2 in, 2 out]
      n45 = property on="RED BAND" class="DigNum (strict)"("Visible"=w16, "Value"=46 ("RED BAND")) -> ()  [unwired: 2 in, 2 out]
      n46 = property on="GREEN BAND" class="DigNum (strict)"("Visible"=w16, "Value"=23 ("GREEN BAND")) -> ()  [unwired: 2 in, 2 out]
      n47 = property on="BLUE BAND" class="DigNum (strict)"("Visible"=w16, "Value"=1 ("BLUE BAND")) -> ()  [unwired: 2 in, 2 out]
      n48 = property on="BAND TO VISUALIZE" class="DigNum (strict)"("Visible"=w16, "Value"=45 ("BAND TO VISUALIZE")) -> ()  [unwired: 2 in, 2 out]
      n49 = property on="RED BAND 2" class="DigNum (strict)"("Visible"=w10, "Value"=46 ("RED BAND")) -> ()  [unwired: 2 in, 2 out]
      n50 = property on="GREEN BAND 2" class="DigNum (strict)"("Visible"=w10, "Value"=23 ("GREEN BAND")) -> ()  [unwired: 2 in, 2 out]
      n51 = property on="BLUE BAND 2" class="DigNum (strict)"("Visible"=w10, "Value"=1 ("BLUE BAND")) -> ()  [unwired: 2 in, 2 out]
      n52 = property on="BAND TO VISUALIZE 2" class="DigNum (strict)"("Visible"=w10, "Value"=45 ("BAND TO VISUALIZE")) -> ()  [unwired: 2 in, 2 out]
      n53 = property on="RED BAND 3" class="DigNum (strict)"("Visible"=w5, "Value"=46 ("RED BAND")) -> ()  [unwired: 2 in, 2 out]
      n54 = property on="GREEN BAND 3" class="DigNum (strict)"("Visible"=w5, "Value"=23 ("GREEN BAND")) -> ()  [unwired: 2 in, 2 out]
      n55 = property on="BLUE BAND 3" class="DigNum (strict)"("Visible"=w5, "Value"=1 ("BLUE BAND")) -> ()  [unwired: 2 in, 2 out]
      n56 = property on="BAND TO VISUALIZE 3" class="DigNum (strict)"("Visible"=w5, "Value"=45 ("BAND TO VISUALIZE")) -> ()  [unwired: 2 in, 2 out]
    }
    frame #1 {
      # "MAIN"
      n57 = while {
        stop <- w44 stop-if-true
        n58 = event shown="[4] \"DEMO\": Mouse Up" {
          selector: _ -> [_ _ _ _ _]
          dyn-events: _ -> [_ _ _ _ _]
          timeout: _ -> [_ _ _ _ _]
          tunnel: [FALSE FALSE FALSE w385 FALSE] -> w44
          event Timeout {
            n59 = event-data() -> ()  [unwired: 1 in, 3 out]
          }
          event "CLUSTERIZATION": Mouse Up {
            # "CLASSIF PAR LOT"
            n60 = event-data() -> ()  [unwired: 1 in, 8 out]
            n61 = stacked-sequence {
              frame #0 {
                w49 = TRUE ("Visible")
                w52 = FALSE
                w55 = T5 0 items=["Grayscale (U8)", "Grayscale (I16)", "Grayscale (SGL)", "Complex (CSG)", "RGB (U32)", "HSL (U32)", "RGB (U64)", "Grayscale (U16)"] ("Image Type")
                w61 = T5 0 items=["Grayscale (U8)", "Grayscale (I16)", "Grayscale (SGL)", "Complex (CSG)", "RGB (U32)", "HSL (U32)", "RGB (U64)", "Grayscale (U16)"] ("Image Type")
                w50 = FALSE ("BACK TO MAIN")
                w53 = TRUE ("Visible")
                w64 = FALSE ("Visible")
                # "INIT"
                n62 = property on="IMAGES FOLDER PATH" class="Path"("Visible"=w53, "DisabledEnum"=T3."Enabled" ("Désactivé"), "Value"=path "" ("IMAGES FOLDER PATH")) -> ()  [unwired: 2 in, 2 out]
                n63 = property on="# Clusters" class="DigNum (strict)"("Visible"=w53) -> ()  [unwired: 2 in, 2 out]
                n64 = property on="# Iterations" class="DigNum (strict)"("Visible"=w53) -> ()  [unwired: 2 in, 2 out]
                n65 = property on="CLUSTER" class="ImageControl"("Visible"=w53) -> ()  [unwired: 2 in, 2 out]
                n66 = property on="BACK TO MAIN" class="Bool (strict)"("Visible"=w53, "Value"=w50) -> ()  [unwired: 2 in, 2 out]
                n67 = property on="DISPLAY 1 BAND" class="ImageControl"("Visible"=w53) -> ()  [unwired: 2 in, 2 out]
                n68 = property on="CURRENT PICTURE ANALYZED" class="Str"("Visible"=w53, "Value"="" ("CURRENT PICTURE ANALYZED")) -> ()  [unwired: 2 in, 2 out]
                n69 = property on="DISPLAY RGB IMAGE" class="ImageControl"("Visible"=w50) -> ()  [unwired: 2 in, 2 out]
                n70 = property on="START CLUSTERIZATION" class="Bool (strict)"("Visible"=w53, "Value"=w50) -> ()  [unwired: 2 in, 2 out]
                n71 = property on="SPECTRA OF CLUSTER CENTERS" class="XYGraph (strict)"("Visible"=w53, "Value"=T4 [] ("SPECTRUM ON ROI")) -> ()  [unwired: 2 in, 2 out]
                n72 = property on="XSTART" class="DigNum (strict)"("Visible"=w49) -> ()  [unwired: 2 in, 2 out]
                n73 = property on="YSTART" class="DigNum (strict)"("Visible"=w49) -> ()  [unwired: 2 in, 2 out]
                n74 = property on="XEND" class="DigNum (strict)"("Visible"=w49) -> ()  [unwired: 2 in, 2 out]
                n75 = property on="YEND" class="DigNum (strict)"("Visible"=w49) -> ()  [unwired: 2 in, 2 out]
                n76 = property on="RED BAND" class="DigNum (strict)"("Visible"=w52) -> ()  [unwired: 2 in, 2 out]
                n77 = property on="GREEN BAND" class="DigNum (strict)"("Visible"=w52) -> ()  [unwired: 2 in, 2 out]
                n78 = property on="BLUE BAND" class="DigNum (strict)"("Visible"=w52) -> ()  [unwired: 2 in, 2 out]
                n79 = property on="BAND TO VISUALIZE" class="DigNum (strict)"("Visible"=TRUE, "Value"=45 ("BAND TO VISUALIZE")) -> ()  [unwired: 2 in, 2 out]
                n80 = property on="QUIT" class="Bool (strict)"("Visible"=w64) -> ()  [unwired: 2 in, 2 out]
                n81 = property on="CLUSTERIZATION" class="Bool (strict)"("Visible"=w64) -> ()  [unwired: 2 in, 2 out]
                n82 = property on="AVERAGE SPECTRUM" class="Bool (strict)"("Visible"=w64) -> ()  [unwired: 2 in, 2 out]
                n83 = property on="DEMO" class="Bool (strict)"("Visible"=w64) -> ()  [unwired: 2 in, 2 out]
                n84 = property on="path" class="Path"("Value"=path "" ("path 2")) -> ()  [unwired: 2 in, 2 out]
                n85 = disable-structure shown="Désactivé" {
                  frame Disabled {
                    w66 = T5 0 items=["Grayscale (U8)", "Grayscale (I16)", "Grayscale (SGL)", "Complex (CSG)", "RGB (U32)", "HSL (U32)", "RGB (U64)", "Grayscale (U16)"] ("Image Type")
                    n86 = call "IMAQ Create"("Image Name"="RGB IMAGE", "Image Type"=w66) -> ("New Image"=w65:T1)  [unwired: 3 in, 1 out]
                    n87 = property on="DISPLAY RGB IMAGE" class="ImageControl"("Value"=w65) -> ()  [unwired: 2 in, 2 out]
                  }
                  frame Enabled {
                  }
                }
                n88 = call "IMAQ Create"("Image Name"="CLUSTER", "Image Type"=w55) -> ("New Image"=w54:T1)  [unwired: 3 in, 1 out]
                n89 = call "IMAQ Create"("Image Name"="VISU 1 LAYER", "Image Type"=w61) -> ("New Image"=w60:T1)  [unwired: 3 in, 1 out]
                n90 = property on="CLUSTER" class="ImageControl"("Value"=w54) -> ()  [unwired: 2 in, 2 out]
                n91 = property on="DISPLAY 1 BAND" class="ImageControl"("Value"=w60) -> ()  [unwired: 2 in, 2 out]
                n92 = property on="VISU 1 LAYER U8" class="IMAQImage (strict)"("Value"=w60) -> ()  [unwired: 2 in, 2 out]
              }
              frame #1 {
                n93 = while {
                  stop <- w68 stop-if-true
                  n94 = event shown="[3] \"IMAGES FOLDER PATH\": Value Change" {
                    selector: _ -> [_ _ _ _ _]
                    dyn-events: _ -> [_ _ _ _ _]
                    timeout: _ -> [_ _ _ _ _]
                    tunnel: [FALSE FALSE FALSE FALSE TRUE] -> w68
                    event Timeout {
                      n95 = event-data() -> ()  [unwired: 1 in, 3 out]
                    }
                    event "START CLUSTERIZATION": Mouse Up {
                      n96 = event-data() -> ()  [unwired: 1 in, 8 out]
                      n97 = property on="IMAGES FOLDER PATH" class="Path"() -> ("Value"=w72:path)  [unwired: 2 in, 2 out]
                      n98 = List Folder(path=w72, pattern="*.hdr" ("filtre")) -> (filenames=w71:string[])  [unwired: 2 in, 3 out]
                      n99 = Array Size(array=w71) -> (size(s)=w74:i32)
                      n100 = Array Size(array=w71) -> (size(s)=w70:i32)
                      n101 = Not Equal To 0?(x=w74) -> (x != 0?=w73:bool)
                      n102 = case shown="True" w73 {
                        tunnel: w71 -> [_ w80]
                        tunnel: w72 -> [_ w79]
                        tunnel: w70 -> [_ w78]
                        frame False {
                          n103 = One Button Dialog(message="No hdr files in the selected folder. Please select another folder ") -> ()  [unwired: 1 in, 1 out]
                        }
                        frame True {
                          n104 = stacked-sequence {
                            tunnel: w80 -> [_ w107 _]
                            tunnel: w79 -> [_ w106 _]
                            tunnel: w78 -> [_ w105 _]
                            frame #0 {
                              w82 = FALSE ("Visible")
                              n105 = property on="BACK TO MAIN" class="Bool (strict)"("Visible"=w82) -> ()  [unwired: 2 in, 2 out]
                              n106 = property on="START CLUSTERIZATION" class="Bool (strict)"("Visible"=w82) -> ()  [unwired: 2 in, 2 out]
                              n107 = disable-structure shown="Désactivé" {
                                frame Disabled {
                                w86 = FALSE
                                n108 = property on="RED BAND" class="DigNum (strict)"("Visible"=w86) -> ()  [unwired: 2 in, 2 out]
                                n109 = property on="GREEN BAND" class="DigNum (strict)"("Visible"=w86) -> ()  [unwired: 2 in, 2 out]
                                n110 = property on="BLUE BAND" class="DigNum (strict)"("Visible"=w86) -> ()  [unwired: 2 in, 2 out]
                                }
                                frame Enabled {
                                }
                              }
                              n111 = property on="BAND TO VISUALIZE" class="DigNum (strict)"("Visible"=FALSE) -> ()  [unwired: 2 in, 2 out]
                              n112 = property on="IMAGES FOLDER PATH" class="Path"("DisabledEnum"=T3."Disabled and Grayed Out" ("Désactivé")) -> ()  [unwired: 2 in, 2 out]
                              n113 = property on="ANALYSIS IN PROGRESS" class="Slide (strict)"("Visible"=TRUE, "Value"=u16 0 ("ANALYSIS IN PROGRESS")) -> ()  [unwired: 2 in, 2 out]
                              n114 = call <vilib>:"Set Busy.vi"() -> ()  [unwired: 10 in, 2 out]
                            }
                            frame #1 {
                              w87 = "\t"
                              n115 = for {
                                tunnel: w107 -> [w131] mode=indexing
                                tunnel: w106 -> [w144]
                                tunnel: w105 -> [w136]
                                shift-right: [w129] -> w102
                                shift-left: string[][] [] -> [w130]
                                i -> [w137]
                                n116 = Build Path(base path=w144, name or relative path=w131) -> (appended path=w117:path)
                                n117 = property on="CURRENT PICTURE ANALYZED" class="Str"("Value"=w131) -> ()  [unwired: 2 in, 2 out]
                                n118 = Increment(x=w137) -> (x+1=w139:i32)
                                n119 = call "extract_wavelength.vi"("Path_image"=w117) -> ("WAVELENGTH"=w127:sgl[])  [unwired: 1 out]
                                n120 = property on="BAND TO VISUALIZE" class="DigNum (strict)"() -> ("Value"=w118:i32)  [unwired: 2 in, 2 out]
                                n121 = Divide(x=w139, y=w136) -> (x/y=w141:dbl)
                                n122 = Multiply(x=w141, y=100.0) -> (x*y=w140:dbl)
                                n123 = call "read_layer.vi"("IMAGE PATH"=w117, "Band"=w118) -> ("Image"=w111:u8[][])  [unwired: 8 in, 1 out]
                                n124 = property on="# Iterations" class="DigNum (strict)"() -> ("Value"=w142:i16)  [unwired: 2 in, 2 out]
                                n125 = Array Size(array=w111) -> (size(s)=w112:i32[])
                                n126 = property on="ANALYSIS IN PROGRESS" class="Slide (strict)"("Value"=w140) -> ()  [unwired: 2 in, 2 out]
                                n127 = property on="# Clusters" class="DigNum (strict)"() -> ("Value"=w124:i16)  [unwired: 2 in, 2 out]
                                n128 = property on="YSTART" class="DigNum (strict)"() -> ("Value"=w115:i16)  [unwired: 2 in, 2 out]
                                n129 = property on="XSTART" class="DigNum (strict)"() -> ("Value"=w116:i16)  [unwired: 2 in, 2 out]
                                n130 = Index Array(array=w112, index=0 ("indice")) -> (element=w109:i32)
                                n131 = Index Array(array=w112, index=1 ("indice")) -> (element=w110:i32)
                                n132 = call "cluster.vi"("IMAGE PATH"=w117, "Nb Iteration"=w142, "YSTART"=w115, "XEND"=w110, "Nb Cluster"=w124, "YEND"=w109, "XSTART"=w116) -> ("CENTRAL SPECTRA"=w121:dbl[][], "CLUSTERS"=w125:i32[][])
                                n133 = property on="YEND" class="DigNum (strict)"("Value"=w109) -> ()  [unwired: 2 in, 2 out]
                                n134 = property on="XEND" class="DigNum (strict)"("Value"=w110) -> ()  [unwired: 2 in, 2 out]
                                n135 = call "cluster_to_image.vi"("CLUSTER"=w125) -> ("Image"=w143:T1)
                                n136 = property on="VISU 1 LAYER U8" class="IMAQImage (strict)"() -> ("Value"=w120:T1)  [unwired: 2 in, 2 out]
                                n137 = property on="CLUSTER" class="ImageControl"("Value"=w143) -> ()  [unwired: 2 in, 2 out]
                                n138 = call "graph_spectrum.vi"("SPECTRUM"=w121, "WAVELENGTH"=w127) -> ("GRAPHE SPECTRUM"=w126:cluster{"WAVELENGTH":dbl[], "SPECTRUM":dbl[]}[])
                                n139 = call "IMAQ ArrayToImage"("Image Pixels (U8)"=w111, "Image"=w120) -> ("Image Out"=w119:T1)  [unwired: 8 in, 1 out]
                                n140 = property on="DISPLAY 1 BAND" class="ImageControl"("Value"=w119) -> ()  [unwired: 2 in, 2 out]
                                n141 = Array Size(array=w121) -> (size(s)=w122:i32[])
                                n142 = property on="SPECTRA OF CLUSTER CENTERS" class="XYGraph (strict)"("Value"=w126) -> ()  [unwired: 2 in, 2 out]
                                n143 = Index Array(array=w122, index=0 ("indice")) -> (element=w108:i32)
                                n144 = Initialize Array(w131, w108) -> (w134:string[])
                                n145 = Number To Fractional String(number=w121, precision (6)=i16 4 ("précision (6)")) -> (F-format string=w123:string[][])  [unwired: 2 in]
                                n146 = Insert Into Array(array=w123, index (col)=0 ("indice désactivé (col)"), new element=w134) -> (w135:string[][])  [unwired: 1 in]
                                n147 = Build Array (concatenate)(w130, w135) -> (w129:string[][])
                              }
                              n148 = property on="WAVELENGTH" class="Arr (strict)"() -> ("Value"=w96:sgl[])  [unwired: 2 in, 2 out]
                              n149 = Array To Spreadsheet String(delimiter (Tab)="\t", array=w102, 3:"%s" ("chaîne de format")) -> (spreadsheet string=w101:string)
                              n150 = Number To Fractional String(number=w96, precision (6)=i16 2 ("précision (6)")) -> (F-format string=w95:string[])  [unwired: 2 in]
                              n151 = Array To Spreadsheet String(delimiter (Tab)="\t", array=w95, 3:"%s" ("chaîne de format")) -> (spreadsheet string=w91:string)
                              n152 = Concatenate Strings("FILENAME", w87, "CLUSTER" ("chaîne"), w87, "AREA" ("chaîne"), w87, w91) -> (w93:string)
                              n153 = Concatenate Strings(w93, w101) -> (w100:string)
                              n154 = Write to Text File(prompt (Choose or enter file path)="please create your spectrum result_file" ("message (sélectionnez ou entrez un chemin de fichier)"), text=w100) -> ()  [unwired: 2 in, 3 out]
                            }
                            frame #2 {
                              w152 = FALSE
                              w155 = TRUE ("Visible")
                              n155 = property on="START CLUSTERIZATION" class="Bool (strict)"("Visible"=w155) -> ()  [unwired: 2 in, 2 out]
                              n156 = property on="BACK TO MAIN" class="Bool (strict)"("Visible"=w155) -> ()  [unwired: 2 in, 2 out]
                              n157 = property on="BAND TO VISUALIZE" class="DigNum (strict)"("Visible"=TRUE) -> ()  [unwired: 2 in, 2 out]
                              n158 = property on="RED BAND" class="DigNum (strict)"("Visible"=w152) -> ()  [unwired: 2 in, 2 out]
                              n159 = property on="GREEN BAND" class="DigNum (strict)"("Visible"=w152) -> ()  [unwired: 2 in, 2 out]
                              n160 = property on="BLUE BAND" class="DigNum (strict)"("Visible"=w152) -> ()  [unwired: 2 in, 2 out]
                              n161 = property on="SPECTRA OF CLUSTER CENTERS" class="XYGraph (strict)"("Value"=T4 [] ("SPECTRUM ON ROI")) -> ()  [unwired: 2 in, 2 out]
                              n162 = call <vilib>:"Unset Busy.vi"() -> ()  [unwired: 11 in, 1 out]
                              n163 = property on="IMAGES FOLDER PATH" class="Path"("DisabledEnum"=T3."Enabled" ("Désactivé")) -> ()  [unwired: 2 in, 2 out]
                              n164 = property on="ANALYSIS IN PROGRESS" class="Slide (strict)"("Value"=u16 0 ("ANALYSIS IN PROGRESS")) -> ()  [unwired: 2 in, 2 out]
                              n165 = call "IMAQ Create"("Image Name"="null") -> ("New Image"=w150:T1)  [unwired: 4 in, 1 out]
                              n166 = call "IMAQ Create"("Image Name"="null") -> ("New Image"=w149:T1)  [unwired: 4 in, 1 out]
                              n167 = property on="DISPLAY 1 BAND" class="ImageControl"("Value"=w150) -> ()  [unwired: 2 in, 2 out]
                              n168 = property on="CLUSTER" class="ImageControl"("Value"=w149) -> ()  [unwired: 2 in, 2 out]
                              n169 = property on="CURRENT PICTURE ANALYZED" class="Str"("Value"="" ("CURRENT PICTURE ANALYZED")) -> ()  [unwired: 2 in, 2 out]
                            }
                          }
                        }
                      }
                    }
                    event "BAND TO VISUALIZE": Value Change {
                      n170 = event-data() -> ()  [unwired: 1 in, 6 out]
                      n171 = property on="path" class="Path"() -> ("Value"=w158:path)  [unwired: 2 in, 2 out]
                      n172 = property on="BAND TO VISUALIZE" class="DigNum (strict)"() -> ("Value"=w157:i32)  [unwired: 2 in, 2 out]
                      n173 = call "read_layer.vi"("IMAGE PATH"=w158, "Band"=w157) -> ("Image"=w156:u8[][])  [unwired: 8 in, 1 out]
                      n174 = property on="VISU 1 LAYER U8" class="IMAQImage (strict)"() -> ("Value"=w161:T1)  [unwired: 2 in, 2 out]
                      n175 = call "IMAQ ArrayToImage"("Image Pixels (U8)"=w156, "Image"=w161) -> ("Image Out"=w160:T1)  [unwired: 8 in, 1 out]
                      n176 = property on="DISPLAY 1 BAND" class="ImageControl"("Value"=w160) -> ()  [unwired: 2 in, 2 out]
                    }
                    event "IMAGES FOLDER PATH": Value Change {
                      n177 = event-data() -> ()  [unwired: 1 in, 6 out]
                      n178 = flat-sequence {
                        frame #0 {
                          n179 = call <vilib>:"Set Busy.vi"() -> ()  [unwired: 10 in, 2 out]
                        }
                        frame #1 {
                          w164 = i16 0 ("XSTART")
                          n180 = property on="IMAGES FOLDER PATH" class="Path"() -> ("Value"=w180:path)  [unwired: 2 in, 2 out]
                          n181 = List Folder(path=w180, pattern="*.hdr" ("filtre")) -> (path out=w172:path, filenames=w174:string[])  [unwired: 2 in, 2 out]
                          n182 = property on="XSTART" class="DigNum (strict)"("Value"=w164) -> ()  [unwired: 2 in, 2 out]
                          n183 = property on="YSTART" class="DigNum (strict)"("Value"=w164) -> ()  [unwired: 2 in, 2 out]
                          n184 = Index Array(array=w174, index=0 ("indice")) -> (element=w173:string)
                          n185 = Build Path(base path=w172, name or relative path=w173) -> (appended path=w163:path)
                          n186 = property on="CURRENT PICTURE ANALYZED" class="Str"("Value"=w173) -> ()  [unwired: 2 in, 2 out]
                          n187 = property on="path" class="Path"("Value"=w163) -> ()  [unwired: 2 in, 2 out]
                          n188 = call "extract_wavelength.vi"("Path_image"=w163) -> ("WAVELENGTH"=w175:sgl[], "WAVELENGTH NUMBER"=w181:i32)
                          n189 = property on="BAND TO VISUALIZE" class="DigNum (strict)"() -> ("Value"=w171:i32)  [unwired: 2 in, 2 out]
                          n190 = property on="WAVELENGTH" class="Arr (strict)"("Value"=w175) -> ()  [unwired: 2 in, 2 out]
                          n191 = property on="WAVELENGTH NUMBER" class="DigNum (strict)"("Value"=w181) -> ()  [unwired: 2 in, 2 out]
                          n192 = call "read_layer.vi"("IMAGE PATH"=w163, "Band"=w171) -> ("Image"=w165:u8[][])  [unwired: 8 in, 1 out]
                          n193 = Array Size(array=w165) -> (size(s)=w168:i32[])
                          n194 = Index Array(array=w168, index=0 ("indice")) -> (element=w167:i32)
                          n195 = Index Array(array=w168, index=1 ("indice")) -> (element=w166:i32)
                          n196 = property on="VISU 1 LAYER U8" class="IMAQImage (strict)"() -> ("Value"=w177:T1)  [unwired: 2 in, 2 out]
                          n197 = property on="YEND" class="DigNum (strict)"("Value"=w167) -> ()  [unwired: 2 in, 2 out]
                          n198 = call "IMAQ ArrayToImage"("Image Pixels (U8)"=w165, "Image"=w177) -> ("Image Out"=w176:T1)  [unwired: 8 in, 1 out]
                          n199 = property on="XEND" class="DigNum (strict)"("Value"=w166) -> ()  [unwired: 2 in, 2 out]
                          n200 = property on="DISPLAY 1 BAND" class="ImageControl"("Value"=w176) -> ()  [unwired: 2 in, 2 out]
                        }
                        frame #2 {
                          n201 = call <vilib>:"Unset Busy.vi"() -> ()  [unwired: 11 in, 1 out]
                        }
                      }
                    }
                    event "BACK TO MAIN": Mouse Up {
                      n202 = event-data() -> ()  [unwired: 1 in, 8 out]
                    }
                  }
                }
              }
              frame #2 {
                w183 = FALSE
                w185 = FALSE
                w187 = FALSE ("QUIT")
                w184 = FALSE ("Visible")
                w188 = TRUE ("Visible")
                n203 = property on="IMAGES FOLDER PATH" class="Path"("Visible"=w184) -> ()  [unwired: 2 in, 2 out]
                n204 = property on="# Clusters" class="DigNum (strict)"("Visible"=w184) -> ()  [unwired: 2 in, 2 out]
                n205 = property on="# Iterations" class="DigNum (strict)"("Visible"=w184) -> ()  [unwired: 2 in, 2 out]
                n206 = property on="CLUSTER" class="ImageControl"("Visible"=w184) -> ()  [unwired: 2 in, 2 out]
                n207 = property on="BACK TO MAIN" class="Bool (strict)"("Visible"=w184, "Value"=w184) -> ()  [unwired: 2 in, 2 out]
                n208 = property on="DISPLAY 1 BAND" class="ImageControl"("Visible"=w184) -> ()  [unwired: 2 in, 2 out]
                n209 = property on="DISPLAY RGB IMAGE" class="ImageControl"("Visible"=w184) -> ()  [unwired: 2 in, 2 out]
                n210 = property on="START CLUSTERIZATION" class="Bool (strict)"("Visible"=w184, "Value"=w184) -> ()  [unwired: 2 in, 2 out]
                n211 = property on="SPECTRA OF CLUSTER CENTERS" class="XYGraph (strict)"("Visible"=w184) -> ()  [unwired: 2 in, 2 out]
                n212 = property on="CURRENT PICTURE ANALYZED" class="Str"("Visible"=w184) -> ()  [unwired: 2 in, 2 out]
                n213 = property on="ANALYSIS IN PROGRESS" class="Slide (strict)"("Visible"=w184) -> ()  [unwired: 2 in, 2 out]
                n214 = property on="BAND TO VISUALIZE" class="DigNum (strict)"("Visible"=w185) -> ()  [unwired: 2 in, 2 out]
                n215 = property on="RED BAND" class="DigNum (strict)"("Visible"=w185) -> ()  [unwired: 2 in, 2 out]
                n216 = property on="GREEN BAND" class="DigNum (strict)"("Visible"=w185) -> ()  [unwired: 2 in, 2 out]
                n217 = property on="BLUE BAND" class="DigNum (strict)"("Visible"=w185) -> ()  [unwired: 2 in, 2 out]
                n218 = property on="QUIT" class="Bool (strict)"("Visible"=w188, "Value"=w187) -> ()  [unwired: 2 in, 2 out]
                n219 = property on="CLUSTERIZATION" class="Bool (strict)"("Visible"=w188, "Value"=w187) -> ()  [unwired: 2 in, 2 out]
                n220 = property on="AVERAGE SPECTRUM" class="Bool (strict)"("Visible"=w188, "Value"=w187) -> ()  [unwired: 2 in, 2 out]
                n221 = property on="DEMO" class="Bool (strict)"("Visible"=w188, "Value"=w187) -> ()  [unwired: 2 in, 2 out]
                n222 = property on="XSTART" class="DigNum (strict)"("Visible"=w183) -> ()  [unwired: 2 in, 2 out]
                n223 = property on="YSTART" class="DigNum (strict)"("Visible"=w183) -> ()  [unwired: 2 in, 2 out]
                n224 = property on="XEND" class="DigNum (strict)"("Visible"=w183) -> ()  [unwired: 2 in, 2 out]
                n225 = property on="YEND" class="DigNum (strict)"("Visible"=w183) -> ()  [unwired: 2 in, 2 out]
                n226 = call "IMAQ Dispose"("All Images? (No)"=TRUE) -> ()  [unwired: 5 in, 1 out]
              }
            }
          }
          event "AVERAGE SPECTRUM": Mouse Up {
            n227 = event-data() -> ()  [unwired: 1 in, 8 out]
            n228 = stacked-sequence {
              frame #0 {
                w197 = TRUE
                w199 = T5 0 items=["Grayscale (U8)", "Grayscale (I16)", "Grayscale (SGL)", "Complex (CSG)", "RGB (U32)", "HSL (U32)", "RGB (U64)", "Grayscale (U16)"] ("Image Type")
                w203 = FALSE ("BACK TO MAIN")
                w207 = T5 0 items=["Grayscale (U8)", "Grayscale (I16)", "Grayscale (SGL)", "Complex (CSG)", "RGB (U32)", "HSL (U32)", "RGB (U64)", "Grayscale (U16)"] ("Image Type")
                w210 = FALSE
                w190 = TRUE
                w204 = FALSE
                # "INIT LOT SPECTRE MOYEN"
                n229 = property on="AVERAGE SPECTRUM" class="Bool (strict)"("Visible"=w204) -> ()  [unwired: 2 in, 2 out]
                n230 = property on="CLUSTERIZATION" class="Bool (strict)"("Visible"=w204) -> ()  [unwired: 2 in, 2 out]
                n231 = property on="DEMO" class="Bool (strict)"("Visible"=w204) -> ()  [unwired: 2 in, 2 out]
                n232 = property on="QUIT" class="Bool (strict)"("Visible"=w204) -> ()  [unwired: 2 in, 2 out]
                n233 = property on="SPECTRA OF CLUSTER CENTERS" class="XYGraph (strict)"("Visible"=w204) -> ()  [unwired: 2 in, 2 out]
                n234 = property on="IMAGES FOLDER" class="Path"("Visible"=w190, "Value"=path "" ("IMAGES FOLDER PATH 2"), "DisabledEnum"=T3."Enabled" ("Désactivé")) -> ()  [unwired: 2 in, 2 out]
                n235 = property on="DISPLAY 1 BAND" class="ImageControl"("Visible"=w190) -> ()  [unwired: 2 in, 2 out]
                n236 = property on="BACK TO MAIN 2" class="Bool (strict)"("Visible"=w190, "Value"=w203) -> ()  [unwired: 2 in, 2 out]
                n237 = property on="CURRENT PICTURE ANALYZED" class="Str"("Visible"=w190, "Value"="" ("IMAGE EN COURS")) -> ()  [unwired: 2 in, 2 out]
                n238 = property on="START SPECTRA CALCULATION" class="Bool (strict)"("Visible"=w190, "Value"=w203) -> ()  [unwired: 2 in, 2 out]
                n239 = property on="ROI AUTO" class="Bool (strict)"("Visible"=w190, "Value"=w203) -> ()  [unwired: 2 in, 2 out]
                n240 = property on="DISPLAY RGB IMAGE" class="ImageControl"("Visible"=w190) -> ()  [unwired: 2 in, 2 out]
                n241 = property on="SPECTRUM ON ROI" class="XYGraph (strict)"("Value"=T4 [] ("SPECTRUM ON ROI"), "Visible"=w190) -> ()  [unwired: 2 in, 2 out]
                n242 = property on="WAVELENGTH" class="Arr (strict)"("Visible"=w210) -> ()  [unwired: 2 in, 2 out]
                n243 = property on="WAVELENGTH NUMBER" class="DigNum (strict)"("Visible"=w210) -> ()  [unwired: 2 in, 2 out]
                n244 = property on="CUBE" class="Arr (strict)"("Visible"=w210) -> ()  [unwired: 2 in, 2 out]
                n245 = property on="DISPLAY 1 BAND" class="ImageControl"("ROI"=T2 {"Global Rectangle"=[], "Contours"=[]}) -> ()  [unwired: 2 in, 2 out]
                n246 = call "IMAQ Create"("Image Name"="RGB IMAGE", "Image Type"=w199) -> ("New Image"=w198:T1)  [unwired: 3 in, 1 out]
                n247 = call "IMAQ Create"("Image Name"="VISU 1 LAYER", "Image Type"=w207) -> ("New Image"=w206:T1)  [unwired: 3 in, 1 out]
                n248 = property on="DISPLAY RGB IMAGE" class="ImageControl"("Value"=w198) -> ()  [unwired: 2 in, 2 out]
                n249 = property on="VISU 1 LAYER U8" class="IMAQImage (strict)"("Value"=w206) -> ()  [unwired: 2 in, 2 out]
                n250 = property on="DISPLAY 1 BAND" class="ImageControl"("Value"=w206) -> ()  [unwired: 2 in, 2 out]
                n251 = property on="BAND TO VISUALIZE 2" class="DigNum (strict)"("Visible"=w197, "Value"=45 ("BAND TO VISUALIZE 2")) -> ()  [unwired: 2 in, 2 out]
                n252 = property on="RED BAND 2" class="DigNum (strict)"("Visible"=w197, "Value"=46 ("RED BAND 2")) -> ()  [unwired: 2 in, 2 out]
                n253 = property on="GREEN BAND 2" class="DigNum (strict)"("Visible"=w197, "Value"=23 ("GREEN BAND 2")) -> ()  [unwired: 2 in, 2 out]
                n254 = property on="BLUE BAND 2" class="DigNum (strict)"("Visible"=w197, "Value"=1 ("BLUE BAND 2")) -> ()  [unwired: 2 in, 2 out]
                n255 = property on="path 2" class="Path"("Value"=path "" ("path 2")) -> ()  [unwired: 2 in, 2 out]
              }
              frame #1 {
                n256 = while {
                  stop <- w211 stop-if-true
                  n257 = event shown="[1] \"START SPECTRA CALCULATION\": Mouse Up" {
                    selector: _ -> [_ _ _ _ _ _ _ _]
                    dyn-events: _ -> [_ _ _ _ _ _ _ _]
                    timeout: _ -> [_ _ _ _ _ _ _ _]
                    tunnel: [FALSE FALSE FALSE FALSE _ _ _ TRUE] -> w211
                    event Timeout {
                      n258 = event-data() -> ()  [unwired: 1 in, 3 out]
                    }
                    event "START SPECTRA CALCULATION": Mouse Up {
                      n259 = event-data() -> ()  [unwired: 1 in, 8 out]
                      n260 = stacked-sequence {
                        frame #0 {
                          w214 = FALSE ("Visible")
                          w222 = FALSE ("Visible")
                          n261 = property on="ROI AUTO" class="Bool (strict)"("Visible"=FALSE) -> ("Value"=w221:bool)  [unwired: 2 in, 2 out]
                          n262 = Not(x=w221) -> (.not. x?=w220:bool)
                          n263 = property on="NEXT IMAGE" class="Bool (strict)"("Visible"=w220, "Value"=FALSE ("NEXT IMAGE")) -> ()  [unwired: 2 in, 2 out]
                          n264 = property on="BACK TO MAIN 2" class="Bool (strict)"("Visible"=w222) -> ()  [unwired: 2 in, 2 out]
                          n265 = property on="START SPECTRA CALCULATION" class="Bool (strict)"("Visible"=w222) -> ()  [unwired: 2 in, 2 out]
                          n266 = property on="ANALYSIS IN PROGRESS" class="Slide (strict)"("Visible"=TRUE, "Value"=u16 0 ("ANALYSIS IN PROGRESS")) -> ()  [unwired: 2 in, 2 out]
                          n267 = property on="BLUE BAND 2" class="DigNum (strict)"("Visible"=w214) -> ()  [unwired: 2 in, 2 out]
                          n268 = property on="BAND TO VISUALIZE 2" class="DigNum (strict)"("Visible"=w214) -> ()  [unwired: 2 in, 2 out]
                          n269 = property on="RED BAND 2" class="DigNum (strict)"("Visible"=w214) -> ()  [unwired: 2 in, 2 out]
                          n270 = property on="GREEN BAND 2" class="DigNum (strict)"("Visible"=w214) -> ()  [unwired: 2 in, 2 out]
                          n271 = property on="IMAGES FOLDER" class="Path"("DisabledEnum"=T3."Disabled and Grayed Out" ("Désactivé")) -> ()  [unwired: 2 in, 2 out]
                        }
                        frame #1 {
                          n272 = property on="DISPLAY 1 BAND" class="ImageControl"() -> ("ROI"=w226:T2)  [unwired: 2 in, 2 out]
                          n273 = property on="IMAGES FOLDER" class="Path"() -> ("Value"=w227:path)  [unwired: 2 in, 2 out]
                          n274 = call "is_roi_empty.vi"("ROI"=w226) -> ("roi empty"=w224:bool)
                          n275 = Empty String/Path?(string/path=w227) -> (empty?=w225:bool)
                          n276 = Not Or(1:w224, 2:w225) -> (0:w223:bool)
                          n277 = case shown="True" w223 {
                            tunnel: w227 -> [_ w232]
                            frame False {
                              n278 = One Button Dialog(message="PLEASE SELECT A FOLDER TO ANALYZE AND/OR DEFINE A ROI BEFORE TO PRESS START") -> ()  [unwired: 1 in, 1 out]
                            }
                            frame True {
                              n279 = List Folder(path=w232, pattern="*.hdr" ("filtre")) -> (path out=w242:path, filenames=w230:string[])  [unwired: 2 in, 2 out]
                              n280 = Array Size(array=w230) -> (size(s)=w231:i32)
                              n281 = for {
                                tunnel: w242 -> [w249]
                                tunnel: w230 -> [w248] mode=indexing
                                shift-right: [w260] -> w239
                                shift-left: string[][] [] -> [w259]
                                tunnel: w231 -> [w257]
                                i -> [w258]
                                n282 = property on="ROI AUTO" class="Bool (strict)"() -> ("Value"=w250:bool)  [unwired: 2 in, 2 out]
                                n283 = Increment(x=w258) -> (x+1=w254:i32)
                                n284 = Divide(x=w254, y=w257) -> (x/y=w256:dbl)
                                n285 = case shown="False" w250 {
                                tunnel: [w264 w311] -> w243
                                tunnel: w249 -> [w267 w310]
                                tunnel: w248 -> [w266 w309]
                                tunnel: [w265 w309] -> w246
                                frame False {
                                n286 = stacked-sequence {
                                tunnel: w267 -> [_ w287 _]
                                tunnel: w266 -> [_ w286 _]
                                tunnel: [_ w286 _] -> w265
                                tunnel: [_ w272 _] -> w264
                                frame #0 {
                                n287 = property on="NEXT IMAGE" class="Bool (strict)"("Value"=FALSE ("NEXT IMAGE"), "DisabledEnum"=T3."Disabled and Grayed Out" ("Désactivé")) -> ()  [unwired: 2 in, 2 out]
                                }
                                frame #1 {
                                n288 = Build Path(base path=w287, name or relative path=w286) -> (appended path=w283:path)
                                n289 = property on="CURRENT PICTURE ANALYZED" class="Str"("Value"=w286) -> ()  [unwired: 2 in, 2 out]
                                n290 = property on="BAND TO VISUALIZE 2" class="DigNum (strict)"() -> ("Value"=w282:i32)  [unwired: 2 in, 2 out]
                                n291 = call "get_cube.vi"("Path_image"=w283) -> ("IMAGE U8"=w279:u8[][][], "CUBE"=w271:sgl[][][])  [unwired: 9 in]
                                n292 = property on="GREEN BAND 2" class="DigNum (strict)"() -> ("Value"=w277:i32)  [unwired: 2 in, 2 out]
                                n293 = property on="BLUE BAND 2" class="DigNum (strict)"() -> ("Value"=w276:i32)  [unwired: 2 in, 2 out]
                                n294 = property on="RED BAND 2" class="DigNum (strict)"() -> ("Value"=w278:i32)  [unwired: 2 in, 2 out]
                                n295 = call "extract_wavelength.vi"("Path_image"=w283) -> ("WAVELENGTH"=w270:sgl[])  [unwired: 1 out]
                                n296 = Index Array(array=w279, index (dim 0)=w282) -> (element=w281:u8[][])  [unwired: 2 in]
                                n297 = Index Array(array=w279, index (dim 0)=w278) -> (element=w275:u8[][])  [unwired: 2 in]
                                n298 = Index Array(array=w279, index (dim 0)=w277) -> (element=w274:u8[][])  [unwired: 2 in]
                                n299 = Index Array(array=w279, index (dim 0)=w276) -> (element=w273:u8[][])  [unwired: 2 in]
                                n300 = property on="VISU 1 LAYER U8" class="IMAQImage (strict)"() -> ("Value"=w280:T1)  [unwired: 2 in, 2 out]
                                n301 = property on="WAVELENGTH" class="Arr (strict)"("Value"=w270) -> ()  [unwired: 2 in, 2 out]
                                n302 = call "IMAQ ArrayToImage"("Image Pixels (U8)"=w281, "Image"=w280) -> ("Image Out"=w285:T1)  [unwired: 8 in, 1 out]
                                n303 = call "color_image.vi"("Blue Plane"=w273, "Green Plane"=w274, "Red plane"=w275) -> ("Color Image"=w284:T1)  [unwired: 8 in]
                                n304 = property on="DISPLAY 1 BAND" class="ImageControl"("Value"=w285) -> ()  [unwired: 2 in, 2 out]
                                n305 = property on="DISPLAY RGB IMAGE" class="ImageControl"("Value"=w284) -> ()  [unwired: 2 in, 2 out]
                                n306 = while {
                                tunnel: [w290] -> w272
                                tunnel: w271 -> [w292]
                                tunnel: w270 -> [w291]
                                stop <- "NEXT IMAGE" stop-if-true
                                n307 = property on="DISPLAY 1 BAND" class="ImageControl"() -> ("ROI"=w293:T2)  [unwired: 2 in, 2 out]
                                n308 = property on="NEXT IMAGE" class="Bool (strict)"("DisabledEnum"=T3."Enabled" ("Disabled")) -> ()  [unwired: 2 in, 2 out]
                                n309 = call "get_average_roi_spectrum.vi"("ROI"=w293, "CUBE"=w292) -> ("SPECTRA"=w290:dbl[][])  [unwired: 1 in]
                                n310 = call "graph_spectrum.vi"("SPECTRUM"=w290, "WAVELENGTH"=w291) -> ("GRAPHE SPECTRUM"=w288:cluster{"WAVELENGTH":dbl[], "SPECTRUM":dbl[]}[])
                                n311 = property on="SPECTRUM ON ROI" class="XYGraph (strict)"("Value"=w288) -> ()  [unwired: 2 in, 2 out]
                                }
                                }
                                frame #2 {
                                n312 = property on="NEXT IMAGE" class="Bool (strict)"("DisabledEnum"=T3."Disabled and Grayed Out" ("Désactivé")) -> ()  [unwired: 2 in, 2 out]
                                }
                                }
                                }
                                frame True {
                                n313 = Build Path(base path=w310, name or relative path=w309) -> (appended path=w296:path)
                                n314 = property on="BAND TO VISUALIZE 2" class="DigNum (strict)"() -> ("Value"=w306:i32)  [unwired: 2 in, 2 out]
                                n315 = property on="CURRENT PICTURE ANALYZED" class="Str"("Value"=w309) -> ()  [unwired: 2 in, 2 out]
                                n316 = call "get_cube.vi"("Path_image"=w296) -> ("IMAGE U8"=w303:u8[][][], "CUBE"=w307:sgl[][][])  [unwired: 9 in]
                                n317 = call "extract_wavelength.vi"("Path_image"=w296) -> ("WAVELENGTH"=w308:sgl[])  [unwired: 1 out]
                                n318 = Index Array(array=w303, index (dim 0)=w306) -> (element=w305:u8[][])  [unwired: 2 in]
                                n319 = property on="DISPLAY 1 BAND" class="ImageControl"() -> ("ROI"=w314:T2)  [unwired: 2 in, 2 out]
                                n320 = property on="VISU 1 LAYER U8" class="IMAQImage (strict)"() -> ("Value"=w313:T1)  [unwired: 2 in, 2 out]
                                n321 = call "IMAQ ArrayToImage"("Image Pixels (U8)"=w305, "Image"=w313) -> ("Image Out"=w312:T1)  [unwired: 8 in, 1 out]
                                n322 = property on="WAVELENGTH" class="Arr (strict)"("Value"=w308) -> ()  [unwired: 2 in, 2 out]
                                n323 = property on="DISPLAY 1 BAND" class="ImageControl"("Value"=w312) -> ()  [unwired: 2 in, 2 out]
                                n324 = call "get_average_roi_spectrum.vi"("ROI"=w314, "CUBE"=w307) -> ("SPECTRA"=w311:dbl[][])  [unwired: 1 in]
                                n325 = property on="RED BAND 2" class="DigNum (strict)"() -> ("Value"=w304:i32)  [unwired: 2 in, 2 out]
                                n326 = property on="GREEN BAND 2" class="DigNum (strict)"() -> ("Value"=w302:i32)  [unwired: 2 in, 2 out]
                                n327 = property on="BLUE BAND 2" class="DigNum (strict)"() -> ("Value"=w301:i32)  [unwired: 2 in, 2 out]
                                n328 = call "graph_spectrum.vi"("SPECTRUM"=w311, "WAVELENGTH"=w308) -> ()  [unwired: 1 out]
                                n329 = Index Array(array=w303, index (dim 0)=w304) -> (element=w300:u8[][])  [unwired: 2 in]
                                n330 = Index Array(array=w303, index (dim 0)=w302) -> (element=w299:u8[][])  [unwired: 2 in]
                                n331 = Index Array(array=w303, index (dim 0)=w301) -> (element=w298:u8[][])  [unwired: 2 in]
                                n332 = call "color_image.vi"("Blue Plane"=w298, "Green Plane"=w299, "Red plane"=w300) -> ("Color Image"=w297:T1)  [unwired: 8 in]
                                n333 = property on="DISPLAY RGB IMAGE" class="ImageControl"("Value"=w297) -> ()  [unwired: 2 in, 2 out]
                                }
                                }
                                n334 = Multiply(x=w256, y=100.0) -> (x*y=w244:dbl)
                                n335 = property on="ANALYSIS IN PROGRESS" class="Slide (strict)"("Value"=w244) -> ()  [unwired: 2 in, 2 out]
                                n336 = Array Size(array=w243) -> (size(s)=w252:i32[])
                                n337 = Index Array(array=w252, index=0 ("indice")) -> (element=w251:i32)
                                n338 = Number To Fractional String(number=w243, precision (6)=i16 4 ("précision (6)")) -> (F-format string=w245:string[][])  [unwired: 2 in]
                                n339 = Initialize Array(w246, w251) -> (w247:string[])
                                n340 = Insert Into Array(array=w245, index (col)=0 ("indice désactivé (col)"), new element=w247) -> (w261:string[][])  [unwired: 1 in]
                                n341 = Build Array (concatenate)(w259, w261) -> (w260:string[][])
                              }
                              n342 = property on="WAVELENGTH" class="Arr (strict)"() -> ("Value"=w240:sgl[])  [unwired: 2 in, 2 out]
                              n343 = Array To Spreadsheet String(delimiter (Tab)="\t", array=w239, 3:"%s" ("chaîne de format")) -> (spreadsheet string=w236:string)
                              n344 = call "header_spectrum_sheet.vi"("WAVELENGTH"=w240) -> ("chaîne concaténée"=w237:string)
                              n345 = Concatenate Strings(w237, w236) -> (w234:string)
                              n346 = Write to Text File(prompt (Choose or enter file path)="please create your spectrum result_file" ("message (sélectionnez ou entrez un chemin de fichier)"), text=w234) -> ()  [unwired: 2 in, 3 out]
                            }
                          }
                        }
                        frame #2 {
                          (unwired) T4 [] ("SPECTRUM ON ROI")
                          w324 = FALSE ("Visible")
                          w322 = TRUE ("Visible")
                          n347 = property on="ROI AUTO" class="Bool (strict)"("Visible"=TRUE, "Value"=FALSE ("ROI AUTO")) -> ()  [unwired: 2 in, 2 out]
                          n348 = property on="BACK TO MAIN 2" class="Bool (strict)"("Visible"=w322) -> ()  [unwired: 2 in, 2 out]
                          n349 = property on="BAND TO VISUALIZE 2" class="DigNum (strict)"("Visible"=w322) -> ()  [unwired: 2 in, 2 out]
                          n350 = property on="START SPECTRA CALCULATION" class="Bool (strict)"("Visible"=w322) -> ()  [unwired: 2 in, 2 out]
                          n351 = property on="BLUE BAND 2" class="DigNum (strict)"("Visible"=w322) -> ()  [unwired: 2 in, 2 out]
                          n352 = property on="RED BAND 2" class="DigNum (strict)"("Visible"=w322) -> ()  [unwired: 2 in, 2 out]
                          n353 = property on="GREEN BAND 2" class="DigNum (strict)"("Visible"=w322) -> ()  [unwired: 2 in, 2 out]
                          n354 = property on="NEXT IMAGE" class="Bool (strict)"("Visible"=w324) -> ()  [unwired: 2 in, 2 out]
                          n355 = property on="ANALYSIS IN PROGRESS" class="Slide (strict)"("Visible"=w324) -> ()  [unwired: 2 in, 2 out]
                          n356 = property on="CURRENT PICTURE ANALYZED" class="Str"("Value"="" ("CURRENT PICTURE ANALYZED")) -> ()  [unwired: 2 in, 2 out]
                          n357 = property on="IMAGES FOLDER" class="Path"("DisabledEnum"=T3."Enabled" ("Désactivé")) -> ()  [unwired: 2 in, 2 out]
                          n358 = property on="ANALYSIS IN PROGRESS" class="Slide (strict)"("Value"=u16 0 ("ANALYSIS IN PROGRESS")) -> ()  [unwired: 2 in, 2 out]
                          n359 = call "IMAQ Create"("Image Name"="null") -> ("New Image"=w321:T1)  [unwired: 4 in, 1 out]
                          n360 = call "IMAQ Create"("Image Name"="null") -> ("New Image"=w320:T1)  [unwired: 4 in, 1 out]
                          n361 = property on="DISPLAY 1 BAND" class="ImageControl"("Value"=w321) -> ()  [unwired: 2 in, 2 out]
                          n362 = property on="DISPLAY RGB IMAGE" class="ImageControl"("Value"=w320) -> ()  [unwired: 2 in, 2 out]
                        }
                      }
                    }
                    event "IMAGES FOLDER": Value Change {
                      n363 = event-data() -> ()  [unwired: 1 in, 6 out]
                      n364 = flat-sequence {
                        frame #0 {
                          n365 = call <vilib>:"Set Busy.vi"() -> ()  [unwired: 10 in, 2 out]
                        }
                        frame #1 {
                          n366 = property on="IMAGES FOLDER" class="Path"() -> ("Value"=w347:path)  [unwired: 2 in, 2 out]
                          n367 = List Folder(path=w347, pattern="*.hdr" ("filtre")) -> (path out=w339:path, filenames=w341:string[])  [unwired: 2 in, 2 out]
                          n368 = Index Array(array=w341, index=0 ("indice")) -> (element=w340:string)
                          n369 = Build Path(base path=w339, name or relative path=w340) -> (appended path=w327:path)
                          n370 = property on="CURRENT PICTURE ANALYZED" class="Str"("Value"=w340) -> ()  [unwired: 2 in, 2 out]
                          n371 = property on="BAND TO VISUALIZE" class="DigNum (strict)"() -> ("Value"=w336:i32)  [unwired: 2 in, 2 out]
                          n372 = property on="path 2" class="Path"("Value"=w327) -> ()  [unwired: 2 in, 2 out]
                          n373 = call "get_cube.vi"("Path_image"=w327) -> ("IMAGE U8"=w334:u8[][][], "CUBE"=w337:sgl[][][])  [unwired: 9 in]
                          n374 = call "extract_wavelength.vi"("Path_image"=w327) -> ("WAVELENGTH"=w342:sgl[], "WAVELENGTH NUMBER"=w348:i32)
                          n375 = property on="CUBE" class="Arr (strict)"("Value"=w337) -> ()  [unwired: 2 in, 2 out]
                          n376 = property on="RED BAND" class="DigNum (strict)"() -> ("Value"=w333:i32)  [unwired: 2 in, 2 out]
                          n377 = property on="GREEN BAND" class="DigNum (strict)"() -> ("Value"=w332:i32)  [unwired: 2 in, 2 out]
                          n378 = property on="BLUE BAND" class="DigNum (strict)"() -> ("Value"=w331:i32)  [unwired: 2 in, 2 out]
                          n379 = property on="WAVELENGTH NUMBER" class="DigNum (strict)"("Value"=w348) -> ()  [unwired: 2 in, 2 out]
                          n380 = property on="IMAGE U8" class="Arr (strict)"("Value"=w334) -> ()  [unwired: 2 in, 2 out]
                          n381 = property on="WAVELENGTH" class="Arr (strict)"("Value"=w342) -> ()  [unwired: 2 in, 2 out]
                          n382 = Index Array(array=w334, index (dim 0)=w332) -> (element=w329:u8[][])  [unwired: 2 in]
                          n383 = Index Array(array=w334, index (dim 0)=w333) -> (element=w330:u8[][])  [unwired: 2 in]
                          n384 = Index Array(array=w334, index (dim 0)=w331) -> (element=w328:u8[][])  [unwired: 2 in]
                          n385 = Index Array(array=w334, index (dim 0)=w336) -> (element=w335:u8[][])  [unwired: 2 in]
                          n386 = call "color_image.vi"("Blue Plane"=w328, "Green Plane"=w329, "Red plane"=w330) -> ("Color Image"=w338:T1)  [unwired: 8 in]
                          n387 = property on="VISU 1 LAYER U8" class="IMAQImage (strict)"() -> ("Value"=w344:T1)  [unwired: 2 in, 2 out]
                          n388 = property on="DISPLAY RGB IMAGE" class="ImageControl"("Value"=w338) -> ()  [unwired: 2 in, 2 out]
                          n389 = call "IMAQ ArrayToImage"("Image Pixels (U8)"=w335, "Image"=w344) -> ("Image Out"=w343:T1)  [unwired: 8 in, 1 out]
                          n390 = property on="DISPLAY 1 BAND" class="ImageControl"("Value"=w343) -> ()  [unwired: 2 in, 2 out]
                        }
                        frame #2 {
                          n391 = call <vilib>:"Unset Busy.vi"() -> ()  [unwired: 11 in, 1 out]
                        }
                      }
                    }
                    event "BAND TO VISUALIZE 2": Value Change {
                      n392 = event-data() -> ()  [unwired: 1 in, 6 out]
                      n393 = property on="BAND TO VISUALIZE 2" class="DigNum (strict)"() -> ("Value"=w350:i32)  [unwired: 2 in, 2 out]
                      n394 = property on="IMAGE U8" class="Arr (strict)"() -> ("Value"=w351:u8[][][])  [unwired: 2 in, 2 out]
                      n395 = Index Array(array=w351, index (dim 0)=w350) -> (element=w349:u8[][])  [unwired: 2 in]
                      n396 = property on="VISU 1 LAYER U8" class="IMAQImage (strict)"() -> ("Value"=w354:T1)  [unwired: 2 in, 2 out]
                      n397 = call "IMAQ ArrayToImage"("Image Pixels (U8)"=w349, "Image"=w354) -> ("Image Out"=w353:T1)  [unwired: 8 in, 1 out]
                      n398 = property on="DISPLAY 1 BAND" class="ImageControl"("Value"=w353) -> ()  [unwired: 2 in, 2 out]
                    }
                    event "RED BAND 2": Value Change {
                      n399 = event-data() -> ()  [unwired: 1 in, 6 out]
                      n400 = property on="IMAGE U8" class="Arr (strict)"() -> ("Value"=w361:u8[][][])  [unwired: 2 in, 2 out]
                      n401 = property on="RED BAND 2" class="DigNum (strict)"() -> ("Value"=w360:i32)  [unwired: 2 in, 2 out]
                      n402 = property on="GREEN BAND 2" class="DigNum (strict)"() -> ("Value"=w359:i32)  [unwired: 2 in, 2 out]
                      n403 = property on="BLUE BAND 2" class="DigNum (strict)"() -> ("Value"=w358:i32)  [unwired: 2 in, 2 out]
                      n404 = Index Array(array=w361, index (dim 0)=w360) -> (element=w357:u8[][])  [unwired: 2 in]
                      n405 = Index Array(array=w361, index (dim 0)=w359) -> (element=w356:u8[][])  [unwired: 2 in]
                      n406 = Index Array(array=w361, index (dim 0)=w358) -> (element=w355:u8[][])  [unwired: 2 in]
                      n407 = call "color_image.vi"("Blue Plane"=w355, "Green Plane"=w356, "Red plane"=w357) -> ("Color Image"=w362:T1)  [unwired: 8 in]
                      n408 = property on="DISPLAY RGB IMAGE" class="ImageControl"("Value"=w362) -> ()  [unwired: 2 in, 2 out]
                    }
                    event "GREEN BAND 2": Value Change {
                      n409 = event-data() -> ()  [unwired: 1 in, 6 out]
                      n410 = property on="IMAGE U8" class="Arr (strict)"() -> ("Value"=w369:u8[][][])  [unwired: 2 in, 2 out]
                      n411 = property on="RED BAND 2" class="DigNum (strict)"() -> ("Value"=w368:i32)  [unwired: 2 in, 2 out]
                      n412 = property on="GREEN BAND 2" class="DigNum (strict)"() -> ("Value"=w367:i32)  [unwired: 2 in, 2 out]
                      n413 = property on="BLUE BAND 2" class="DigNum (strict)"() -> ("Value"=w366:i32)  [unwired: 2 in, 2 out]
                      n414 = Index Array(array=w369, index (dim 0)=w368) -> (element=w365:u8[][])  [unwired: 2 in]
                      n415 = Index Array(array=w369, index (dim 0)=w367) -> (element=w364:u8[][])  [unwired: 2 in]
                      n416 = Index Array(array=w369, index (dim 0)=w366) -> (element=w363:u8[][])  [unwired: 2 in]
                      n417 = call "color_image.vi"("Blue Plane"=w363, "Green Plane"=w364, "Red plane"=w365) -> ("Color Image"=w370:T1)  [unwired: 8 in]
                      n418 = property on="DISPLAY RGB IMAGE" class="ImageControl"("Value"=w370) -> ()  [unwired: 2 in, 2 out]
                    }
                    event "BLUE BAND 2": Value Change {
                      n419 = event-data() -> ()  [unwired: 1 in, 6 out]
                      n420 = property on="IMAGE U8" class="Arr (strict)"() -> ("Value"=w377:u8[][][])  [unwired: 2 in, 2 out]
                      n421 = property on="RED BAND 2" class="DigNum (strict)"() -> ("Value"=w376:i32)  [unwired: 2 in, 2 out]
                      n422 = property on="GREEN BAND 2" class="DigNum (strict)"() -> ("Value"=w375:i32)  [unwired: 2 in, 2 out]
                      n423 = property on="BLUE BAND 2" class="DigNum (strict)"() -> ("Value"=w374:i32)  [unwired: 2 in, 2 out]
                      n424 = Index Array(array=w377, index (dim 0)=w376) -> (element=w373:u8[][])  [unwired: 2 in]
                      n425 = Index Array(array=w377, index (dim 0)=w375) -> (element=w372:u8[][])  [unwired: 2 in]
                      n426 = Index Array(array=w377, index (dim 0)=w374) -> (element=w371:u8[][])  [unwired: 2 in]
                      n427 = call "color_image.vi"("Blue Plane"=w371, "Green Plane"=w372, "Red plane"=w373) -> ("Color Image"=w378:T1)  [unwired: 8 in]
                      n428 = property on="DISPLAY RGB IMAGE" class="ImageControl"("Value"=w378) -> ()  [unwired: 2 in, 2 out]
                    }
                    event "BACK TO MAIN 2": Mouse Up {
                      n429 = event-data() -> ()  [unwired: 1 in, 8 out]
                    }
                  }
                }
              }
              frame #2 {
                w381 = FALSE
                w380 = FALSE ("Visible")
                w383 = TRUE ("Visible")
                n430 = property on="CLUSTERIZATION" class="Bool (strict)"("Visible"=w383) -> ()  [unwired: 2 in, 2 out]
                n431 = property on="DEMO" class="Bool (strict)"("Visible"=w383) -> ()  [unwired: 2 in, 2 out]
                n432 = property on="QUIT" class="Bool (strict)"("Visible"=w383) -> ()  [unwired: 2 in, 2 out]
                n433 = property on="AVERAGE SPECTRUM" class="Bool (strict)"("Visible"=w383) -> ()  [unwired: 2 in, 2 out]
                n434 = property on="SPECTRA OF CLUSTER CENTERS" class="XYGraph (strict)"("Visible"=w380) -> ()  [unwired: 2 in, 2 out]
                n435 = property on="IMAGES FOLDER" class="Path"("Visible"=w380) -> ()  [unwired: 2 in, 2 out]
                n436 = property on="ROI AUTO" class="Bool (strict)"("Visible"=w380) -> ()  [unwired: 2 in, 2 out]
                n437 = property on="BACK TO MAIN 2" class="Bool (strict)"("Visible"=w380, "Value"=w380) -> ()  [unwired: 2 in, 2 out]
                n438 = property on="CURRENT PICTURE ANALYZED" class="Str"("Visible"=w380) -> ()  [unwired: 2 in, 2 out]
                n439 = property on="DISPLAY 1 BAND" class="ImageControl"("Visible"=w380) -> ()  [unwired: 2 in, 2 out]
                n440 = property on="START SPECTRA CALCULATION" class="Bool (strict)"("Visible"=w380, "Value"=w380) -> ()  [unwired: 2 in, 2 out]
                n441 = property on="ANALYSIS IN PROGRESS" class="Slide (strict)"("Visible"=w380) -> ()  [unwired: 2 in, 2 out]
                n442 = property on="SPECTRUM ON ROI" class="XYGraph (strict)"("Visible"=w380) -> ()  [unwired: 2 in, 2 out]
                n443 = property on="DISPLAY RGB IMAGE" class="ImageControl"("Visible"=w380) -> ()  [unwired: 2 in, 2 out]
                n444 = property on="BAND TO VISUALIZE 2" class="DigNum (strict)"("Visible"=w381) -> ()  [unwired: 2 in, 2 out]
                n445 = property on="RED BAND 2" class="DigNum (strict)"("Visible"=w381) -> ()  [unwired: 2 in, 2 out]
                n446 = property on="GREEN BAND 2" class="DigNum (strict)"("Visible"=w381) -> ()  [unwired: 2 in, 2 out]
                n447 = property on="BLUE BAND 2" class="DigNum (strict)"("Visible"=w381) -> ()  [unwired: 2 in, 2 out]
                n448 = call "IMAQ Dispose"("All Images? (No)"=TRUE) -> ()  [unwired: 5 in, 1 out]
              }
            }
          }
          event "QUIT": Mouse Up {
            n449 = event-data() -> ()  [unwired: 1 in, 8 out]
            n450 = Two Button Dialog(message="Do you really want to quit ?") -> (T button?=w385:bool)  [unwired: 2 in]
          }
          event "DEMO": Mouse Up {
            n451 = event-data() -> ()  [unwired: 1 in, 8 out]
            n452 = stacked-sequence {
              frame #0 {
                w394 = TRUE
                w395 = TRUE
                w397 = T5 0 items=["Grayscale (U8)", "Grayscale (I16)", "Grayscale (SGL)", "Complex (CSG)", "RGB (U32)", "HSL (U32)", "RGB (U64)", "Grayscale (U16)"] ("Image Type")
                w400 = T5 0 items=["Grayscale (U8)", "Grayscale (I16)", "Grayscale (SGL)", "Complex (CSG)", "RGB (U32)", "HSL (U32)", "RGB (U64)", "Grayscale (U16)"] ("Image Type")
                w404 = T5 0 items=["Grayscale (U8)", "Grayscale (I16)", "Grayscale (SGL)", "Complex (CSG)", "RGB (U32)", "HSL (U32)", "RGB (U64)", "Grayscale (U16)"] ("Image Type")
                w408 = FALSE
                w410 = TRUE
                w411 = FALSE ("ROI Tool Buttons Visible:Annulus Tool Button Visible")
                w393 = TRUE ("Visible")
                n453 = property on="DISPLAY RGB IMAGE" class="ImageControl"("Visible"=w393) -> ()  [unwired: 2 in, 2 out]
                n454 = property on="CLUSTER" class="ImageControl"("Visible"=w393) -> ()  [unwired: 2 in, 2 out]
                n455 = property on="DISPLAY 1 BAND" class="ImageControl"("Visible"=w393) -> ()  [unwired: 2 in, 2 out]
                n456 = property on="IMAGE PATH" class="Path"("Visible"=w393, "Value"=path "" ("IMAGES PATH")) -> ()  [unwired: 2 in, 2 out]
                n457 = property on="BAND TO VISUALIZE 3" class="DigNum (strict)"("Visible"=w393, "Value"=45 ("BAND TO VISUALIZE 3")) -> ()  [unwired: 2 in, 2 out]
                n458 = property on="BACK TO MAIN 3" class="Bool (strict)"("Visible"=w393, "Value"=FALSE ("BACK TO MAIN")) -> ()  [unwired: 2 in, 2 out]
                n459 = property on="CALCULATE CLUSTER" class="Bool (strict)"("Visible"=FALSE, "Value"=FALSE ("CALCULATE CLUSTER")) -> ()  [unwired: 2 in, 2 out]
                n460 = property on="RED BAND 3" class="DigNum (strict)"("Visible"=w394, "Value"=46 ("RED BAND 3")) -> ()  [unwired: 2 in, 2 out]
                n461 = property on="GREEN BAND 3" class="DigNum (strict)"("Visible"=w394, "Value"=23 ("GREEN BAND 3")) -> ()  [unwired: 2 in, 2 out]
                n462 = property on="BLUE BAND 3" class="DigNum (strict)"("Visible"=w394, "Value"=1 ("BLUE BAND 3")) -> ()  [unwired: 2 in, 2 out]
                n463 = property on="DISPLAY 1 BAND" class="ImageControl"("Annulus Tool Button Visible"=w411, "Closed Freehand Tool Button Visible"=w411, "Ellipse Tool Button Visible"=w411, "Freehand Tool Button Visible"=w411, "Line Tool Button Visible"=w411, "Pan Tool Button Visible"=w411, "Polygon Tool Button Visible"=w411, "Polyline Tool Button Visible"=w411, "Rotated Rectangle Tool Button Visible"=w411) -> ()  [unwired: 2 in, 2 out]
                n464 = property on="DISPLAY 1 BAND" class="ImageControl"("ROI"=T2 {"Global Rectangle"=[], "Contours"=[]}) -> ()  [unwired: 2 in, 2 out]
                n465 = property on="SPECTRUM ON ROI" class="XYGraph (strict)"("Value"=T4 [] ("Graphe XY"), "Visible"=TRUE) -> ()  [unwired: 2 in, 2 out]
                n466 = call "IMAQ Create"("Image Name"="CLUSTER", "Image Type"=w397) -> ("New Image"=w396:T1)  [unwired: 3 in, 1 out]
                n467 = call "IMAQ Create"("Image Name"="RGB IMAGE", "Image Type"=w400) -> ("New Image"=w399:T1)  [unwired: 3 in, 1 out]
                n468 = property on="# Iterations" class="DigNum (strict)"("Visible"=w395) -> ()  [unwired: 2 in, 2 out]
                n469 = property on="# Clusters" class="DigNum (strict)"("Visible"=w395) -> ()  [unwired: 2 in, 2 out]
                n470 = property on="XEND" class="DigNum (strict)"("Visible"=w410) -> ()  [unwired: 2 in, 2 out]
                n471 = property on="XSTART" class="DigNum (strict)"("Visible"=w410) -> ()  [unwired: 2 in, 2 out]
                n472 = property on="YEND" class="DigNum (strict)"("Visible"=w410) -> ()  [unwired: 2 in, 2 out]
                n473 = property on="YSTART" class="DigNum (strict)"("Visible"=w410) -> ()  [unwired: 2 in, 2 out]
                n474 = property on="CLUSTER" class="ImageControl"("Value"=w396) -> ()  [unwired: 2 in, 2 out]
                n475 = call "IMAQ Create"("Image Name"="VISU 1 LAYER", "Image Type"=w404) -> ("New Image"=w403:T1)  [unwired: 3 in, 1 out]
                n476 = property on="DISPLAY RGB IMAGE" class="ImageControl"("Value"=w399) -> ()  [unwired: 2 in, 2 out]
                n477 = property on="DISPLAY 1 BAND" class="ImageControl"("Value"=w403) -> ()  [unwired: 2 in, 2 out]
                n478 = property on="VISU 1 LAYER U8" class="IMAQImage (strict)"("Value"=w403) -> ()  [unwired: 2 in, 2 out]
                n479 = property on="AVERAGE SPECTRUM" class="Bool (strict)"("Visible"=w408) -> ()  [unwired: 2 in, 2 out]
                n480 = property on="CLUSTERIZATION" class="Bool (strict)"("Visible"=w408) -> ()  [unwired: 2 in, 2 out]
                n481 = property on="DEMO" class="Bool (strict)"("Visible"=w408) -> ()  [unwired: 2 in, 2 out]
                n482 = property on="QUIT" class="Bool (strict)"("Visible"=w408) -> ()  [unwired: 2 in, 2 out]
              }
              frame #1 {
                n483 = while {
                  stop <- w413 stop-if-true
                  n484 = event shown="[2] \"DISPLAY 1 BAND\": Mouse Up" {
                    selector: _ -> [_ _ _ _ _ _ _ _ _]
                    dyn-events: _ -> [_ _ _ _ _ _ _ _ _]
                    timeout: _ -> [_ _ _ _ _ _ _ _ _]
                    tunnel: [FALSE TRUE FALSE FALSE FALSE _ _ _ FALSE] -> w413
                    event Timeout {
                      n485 = event-data() -> ()  [unwired: 1 in, 3 out]
                    }
                    event "BACK TO MAIN 3": Mouse Up {
                      n486 = event-data() -> ()  [unwired: 1 in, 8 out]
                    }
                    event "DISPLAY 1 BAND": Mouse Up {
                      n487 = event-data() -> ()  [unwired: 1 in, 8 out]
                      n488 = property on="DISPLAY 1 BAND" class="ImageControl"() -> ("ROI"=w419:T2)  [unwired: 2 in, 2 out]
                      n489 = property on="CUBE" class="Arr (strict)"() -> ("Value"=w417:sgl[][][])  [unwired: 2 in, 2 out]
                      n490 = call "get_average_roi_spectrum.vi"("ROI"=w419, "CUBE"=w417) -> ("SPECTRA"=w421:dbl[][])  [unwired: 1 in]
                      n491 = property on="WAVELENGTH" class="Arr (strict)"() -> ("Value"=w420:sgl[])  [unwired: 2 in, 2 out]
                      n492 = call "graph_spectrum.vi"("SPECTRUM"=w421, "WAVELENGTH"=w420) -> ("GRAPHE SPECTRUM"=w416:cluster{"WAVELENGTH":dbl[], "SPECTRUM":dbl[]}[])
                      n493 = property on="SPECTRUM ON ROI" class="XYGraph (strict)"("Value"=w416) -> ()  [unwired: 2 in, 2 out]
                    }
                    event "BAND TO VISUALIZE 3": Value Change {
                      n494 = event-data() -> ()  [unwired: 1 in, 6 out]
                      n495 = property on="BAND TO VISUALIZE 3" class="DigNum (strict)"() -> ("Value"=w423:i32)  [unwired: 2 in, 2 out]
                      n496 = property on="IMAGE U8" class="Arr (strict)"() -> ("Value"=w424:u8[][][])  [unwired: 2 in, 2 out]
                      n497 = Index Array(array=w424, index (dim 0)=w423) -> (element=w422:u8[][])  [unwired: 2 in]
                      n498 = property on="VISU 1 LAYER U8" class="IMAQImage (strict)"() -> ("Value"=w427:T1)  [unwired: 2 in, 2 out]
                      n499 = call "IMAQ ArrayToImage"("Image Pixels (U8)"=w422, "Image"=w427) -> ("Image Out"=w426:T1)  [unwired: 8 in, 1 out]
                      n500 = property on="DISPLAY 1 BAND" class="ImageControl"("Value"=w426) -> ()  [unwired: 2 in, 2 out]
                    }
                    event "IMAGE PATH": Value Change {
                      n501 = event-data() -> ()  [unwired: 1 in, 6 out]
                      n502 = flat-sequence {
                        frame #0 {
                          n503 = call <vilib>:"Set Busy.vi"() -> ()  [unwired: 10 in, 2 out]
                        }
                        frame #1 {
                          w450 = i16 0 ("XSTART")
                          n504 = property on="IMAGE PATH" class="Path"() -> ("Value"=w433:path)  [unwired: 2 in, 2 out]
                          n505 = Strip Path(path=w433) -> (name=w453:string)  [unwired: 1 out]
                          n506 = property on="CALCULATE CLUSTER" class="Bool (strict)"("Visible"=TRUE, "Value"=FALSE ("CALCULATE CLUSTER")) -> ()  [unwired: 2 in, 2 out]
                          n507 = property on="CURRENT PICTURE ANALYZED" class="Str"("Value"=w453) -> ()  [unwired: 2 in, 2 out]
                          n508 = call "extract_wavelength.vi"("Path_image"=w433) -> ("WAVELENGTH"=w452:sgl[], "WAVELENGTH NUMBER"=w445:i32)
                          n509 = property on="BAND TO VISUALIZE 3" class="DigNum (strict)"() -> ("Value"=w441:i32)  [unwired: 2 in, 2 out]
                          n510 = property on="RED BAND 3" class="DigNum (strict)"() -> ("Value"=w439:i32)  [unwired: 2 in, 2 out]
                          n511 = property on="GREEN BAND 3" class="DigNum (strict)"() -> ("Value"=w438:i32)  [unwired: 2 in, 2 out]
                          n512 = property on="BLUE BAND 3" class="DigNum (strict)"() -> ("Value"=w437:i32)  [unwired: 2 in, 2 out]
                          n513 = property on="WAVELENGTH NUMBER" class="DigNum (strict)"("Value"=w445) -> ()  [unwired: 2 in, 2 out]
                          n514 = property on="WAVELENGTH" class="Arr (strict)"("Value"=w452) -> ()  [unwired: 2 in, 2 out]
                          n515 = call "get_cube.vi"("Path_image"=w433) -> ("IMAGE U8"=w432:u8[][][], "CUBE"=w442:sgl[][][])  [unwired: 9 in]
                          n516 = Index Array(array=w432, index (dim 0)=w439) -> (element=w436:u8[][])  [unwired: 2 in]
                          n517 = Index Array(array=w432, index (dim 0)=w438) -> (element=w435:u8[][])  [unwired: 2 in]
                          n518 = Index Array(array=w432, index (dim 0)=w441) -> (element=w440:u8[][])  [unwired: 2 in]
                          n519 = Index Array(array=w432, index (dim 0)=w437) -> (element=w434:u8[][])  [unwired: 2 in]
                          n520 = property on="IMAGE U8" class="Arr (strict)"("Value"=w432) -> ()  [unwired: 2 in, 2 out]
                          n521 = property on="CUBE" class="Arr (strict)"("Value"=w442) -> ()  [unwired: 2 in, 2 out]
                          n522 = call "color_image.vi"("Blue Plane"=w434, "Green Plane"=w435, "Red plane"=w436) -> ("Color Image"=w443:T1)  [unwired: 8 in]
                          n523 = Array Size(array=w432) -> (size(s)=w431:i32[])
                          n524 = property on="VISU 1 LAYER U8" class="IMAQImage (strict)"() -> ("Value"=w446:T1)  [unwired: 2 in, 2 out]
                          n525 = Index Array(array=w431, index=2 ("indice")) -> (element=w429:i32)
                          n526 = call "IMAQ ArrayToImage"("Image Pixels (U8)"=w440, "Image"=w446) -> ("Image Out"=w444:T1)  [unwired: 8 in, 1 out]
                          n527 = Index Array(array=w431, index=1 ("indice")) -> (element=w430:i32)
                          n528 = property on="XEND" class="DigNum (strict)"("Value"=w429) -> ()  [unwired: 2 in, 2 out]
                          n529 = property on="XSTART" class="DigNum (strict)"("Value"=w450) -> ()  [unwired: 2 in, 2 out]
                          n530 = property on="DISPLAY 1 BAND" class="ImageControl"("Value"=w444) -> ()  [unwired: 2 in, 2 out]
                          n531 = property on="YSTART" class="DigNum (strict)"("Value"=w450) -> ()  [unwired: 2 in, 2 out]
                          n532 = property on="DISPLAY RGB IMAGE" class="ImageControl"("Value"=w443) -> ()  [unwired: 2 in, 2 out]
                          n533 = property on="YEND" class="DigNum (strict)"("Value"=w430) -> ()  [unwired: 2 in, 2 out]
                        }
                        frame #2 {
                          n534 = call <vilib>:"Unset Busy.vi"() -> ()  [unwired: 11 in, 1 out]
                        }
                      }
                    }
                    event "RED BAND 3": Value Change {
                      n535 = event-data() -> ()  [unwired: 1 in, 6 out]
                      n536 = property on="IMAGE U8" class="Arr (strict)"() -> ("Value"=w460:u8[][][])  [unwired: 2 in, 2 out]
                      n537 = property on="RED BAND 3" class="DigNum (strict)"() -> ("Value"=w459:i32)  [unwired: 2 in, 2 out]
                      n538 = property on="GREEN BAND 3" class="DigNum (strict)"() -> ("Value"=w458:i32)  [unwired: 2 in, 2 out]
                      n539 = property on="BLUE BAND 3" class="DigNum (strict)"() -> ("Value"=w457:i32)  [unwired: 2 in, 2 out]
                      n540 = Index Array(array=w460, index (dim 0)=w459) -> (element=w456:u8[][])  [unwired: 2 in]
                      n541 = Index Array(array=w460, index (dim 0)=w458) -> (element=w455:u8[][])  [unwired: 2 in]
                      n542 = Index Array(array=w460, index (dim 1)=w457) -> (element=w454:u8[][])  [unwired: 2 in]
                      n543 = call "color_image.vi"("Blue Plane"=w454, "Green Plane"=w455, "Red plane"=w456) -> ("Color Image"=w461:T1)  [unwired: 8 in]
                      n544 = property on="DISPLAY RGB IMAGE" class="ImageControl"("Value"=w461) -> ()  [unwired: 2 in, 2 out]
                    }
                    event "GREEN BAND 3": Value Change {
                      n545 = event-data() -> ()  [unwired: 1 in, 6 out]
                      n546 = property on="IMAGE U8" class="Arr (strict)"() -> ("Value"=w468:u8[][][])  [unwired: 2 in, 2 out]
                      n547 = property on="RED BAND 3" class="DigNum (strict)"() -> ("Value"=w467:i32)  [unwired: 2 in, 2 out]
                      n548 = property on="GREEN BAND 3" class="DigNum (strict)"() -> ("Value"=w466:i32)  [unwired: 2 in, 2 out]
                      n549 = property on="BLUE BAND 3" class="DigNum (strict)"() -> ("Value"=w465:i32)  [unwired: 2 in, 2 out]
                      n550 = Index Array(array=w468, index (dim 0)=w467) -> (element=w464:u8[][])  [unwired: 2 in]
                      n551 = Index Array(array=w468, index (dim 0)=w466) -> (element=w463:u8[][])  [unwired: 2 in]
                      n552 = Index Array(array=w468, index (dim 1)=w465) -> (element=w462:u8[][])  [unwired: 2 in]
                      n553 = call "color_image.vi"("Blue Plane"=w462, "Green Plane"=w463, "Red plane"=w464) -> ("Color Image"=w469:T1)  [unwired: 8 in]
                      n554 = property on="DISPLAY RGB IMAGE" class="ImageControl"("Value"=w469) -> ()  [unwired: 2 in, 2 out]
                    }
                    event "BLUE BAND 3": Value Change {
                      n555 = event-data() -> ()  [unwired: 1 in, 6 out]
                      n556 = property on="IMAGE U8" class="Arr (strict)"() -> ("Value"=w476:u8[][][])  [unwired: 2 in, 2 out]
                      n557 = property on="RED BAND 3" class="DigNum (strict)"() -> ("Value"=w475:i32)  [unwired: 2 in, 2 out]
                      n558 = property on="GREEN BAND 3" class="DigNum (strict)"() -> ("Value"=w474:i32)  [unwired: 2 in, 2 out]
                      n559 = property on="BLUE BAND 3" class="DigNum (strict)"() -> ("Value"=w473:i32)  [unwired: 2 in, 2 out]
                      n560 = Index Array(array=w476, index (dim 0)=w475) -> (element=w472:u8[][])  [unwired: 2 in]
                      n561 = Index Array(array=w476, index (dim 0)=w474) -> (element=w471:u8[][])  [unwired: 2 in]
                      n562 = Index Array(array=w476, index (dim 1)=w473) -> (element=w470:u8[][])  [unwired: 2 in]
                      n563 = call "color_image.vi"("Blue Plane"=w470, "Green Plane"=w471, "Red plane"=w472) -> ("Color Image"=w477:T1)  [unwired: 8 in]
                      n564 = property on="DISPLAY RGB IMAGE" class="ImageControl"("Value"=w477) -> ()  [unwired: 2 in, 2 out]
                    }
                    event "CALCULATE CLUSTER": Mouse Up {
                      n565 = event-data() -> ()  [unwired: 1 in, 8 out]
                      n566 = flat-sequence {
                        frame #0 {
                          n567 = call <vilib>:"Set Busy.vi"() -> ()  [unwired: 10 in, 2 out]
                        }
                        frame #1 {
                          n568 = property on="# Iterations" class="DigNum (strict)"() -> ("Value"=w484:i16)  [unwired: 2 in, 2 out]
                          n569 = property on="IMAGE PATH" class="Path"() -> ("Value"=w486:path)  [unwired: 2 in, 2 out]
                          n570 = property on="XSTART" class="DigNum (strict)"() -> ("Value"=w485:i16)  [unwired: 2 in, 2 out]
                          n571 = property on="YSTART" class="DigNum (strict)"() -> ("Value"=w487:i16)  [unwired: 2 in, 2 out]
                          n572 = property on="XEND" class="DigNum (strict)"() -> ("Value"=w488:i16)  [unwired: 2 in, 2 out]
                          n573 = property on="YEND" class="DigNum (strict)"() -> ("Value"=w489:i16)  [unwired: 2 in, 2 out]
                          n574 = property on="# Clusters" class="DigNum (strict)"() -> ("Value"=w480:i16)  [unwired: 2 in, 2 out]
                          n575 = property on="WAVELENGTH" class="Arr (strict)"() -> ("Value"=w481:sgl[])  [unwired: 2 in, 2 out]
                          n576 = call "cluster.vi"("IMAGE PATH"=w486, "Nb Iteration"=w484, "YSTART"=w487, "XEND"=w488, "Nb Cluster"=w480, "YEND"=w489, "XSTART"=w485) -> ("CENTRAL SPECTRA"=w479:dbl[][], "CLUSTERS"=w483:i32[][])
                          n577 = call "graph_spectrum.vi"("SPECTRUM"=w479, "WAVELENGTH"=w481) -> ("GRAPHE SPECTRUM"=w482:cluster{"WAVELENGTH":dbl[], "SPECTRUM":dbl[]}[])
                          n578 = call "cluster_to_image.vi"("CLUSTER"=w483) -> ("Image"=w490:T1)
                          n579 = property on="CLUSTER" class="ImageControl"("Value"=w490) -> ()  [unwired: 2 in, 2 out]
                          n580 = property on="SPECTRA OF CLUSTER CENTERS" class="XYGraph (strict)"("Value"=w482) -> ()  [unwired: 2 in, 2 out]
                        }
                        frame #2 {
                          n581 = call <vilib>:"Unset Busy.vi"() -> ()  [unwired: 11 in, 1 out]
                        }
                      }
                    }
                  }
                }
              }
              frame #2 {
                w492 = FALSE
                w493 = FALSE
                w497 = TRUE
                w494 = FALSE
                w491 = FALSE ("Visible")
                n582 = property on="DISPLAY RGB IMAGE" class="ImageControl"("Visible"=w491) -> ()  [unwired: 2 in, 2 out]
                n583 = property on="CLUSTER" class="ImageControl"("Visible"=w491) -> ()  [unwired: 2 in, 2 out]
                n584 = property on="CALCULATE CLUSTER" class="Bool (strict)"("Visible"=w491) -> ()  [unwired: 2 in, 2 out]
                n585 = property on="DISPLAY 1 BAND" class="ImageControl"("Visible"=w491) -> ()  [unwired: 2 in, 2 out]
                n586 = property on="BAND TO VISUALIZE 3" class="DigNum (strict)"("Visible"=w491) -> ()  [unwired: 2 in, 2 out]
                n587 = property on="CURRENT PICTURE ANALYZED" class="Str"("Visible"=w491) -> ()  [unwired: 2 in, 2 out]
                n588 = property on="SPECTRUM ON ROI" class="XYGraph (strict)"("Visible"=w491) -> ()  [unwired: 2 in, 2 out]
                n589 = property on="BACK TO MAIN 3" class="Bool (strict)"("Visible"=w491, "Value"=w491) -> ()  [unwired: 2 in, 2 out]
                n590 = property on="IMAGE PATH" class="Path"("Visible"=w491, "Value"=path "" ("IMAGES FOLDER PATH")) -> ()  [unwired: 2 in, 2 out]
                n591 = property on="XSTART" class="DigNum (strict)"("Visible"=w494) -> ()  [unwired: 2 in, 2 out]
                n592 = property on="YEND" class="DigNum (strict)"("Visible"=w494) -> ()  [unwired: 2 in, 2 out]
                n593 = property on="YSTART" class="DigNum (strict)"("Visible"=w494) -> ()  [unwired: 2 in, 2 out]
                n594 = property on="# Iterations" class="DigNum (strict)"("Visible"=w493) -> ()  [unwired: 2 in, 2 out]
                n595 = property on="# Clusters" class="DigNum (strict)"("Visible"=w493) -> ()  [unwired: 2 in, 2 out]
                n596 = property on="XEND" class="DigNum (strict)"("Visible"=w494) -> ()  [unwired: 2 in, 2 out]
                n597 = property on="RED BAND 3" class="DigNum (strict)"("Visible"=w492) -> ()  [unwired: 2 in, 2 out]
                n598 = property on="GREEN BAND 3" class="DigNum (strict)"("Visible"=w492) -> ()  [unwired: 2 in, 2 out]
                n599 = property on="BLUE BAND 3" class="DigNum (strict)"("Visible"=w492) -> ()  [unwired: 2 in, 2 out]
                n600 = property on="AVERAGE SPECTRUM" class="Bool (strict)"("Visible"=w497) -> ()  [unwired: 2 in, 2 out]
                n601 = property on="CLUSTERIZATION" class="Bool (strict)"("Visible"=w497) -> ()  [unwired: 2 in, 2 out]
                n602 = property on="DEMO" class="Bool (strict)"("Visible"=w497) -> ()  [unwired: 2 in, 2 out]
                n603 = property on="QUIT" class="Bool (strict)"("Visible"=w497) -> ()  [unwired: 2 in, 2 out]
                n604 = call "IMAQ Dispose"("All Images? (No)"=TRUE) -> ()  [unwired: 5 in, 1 out]
              }
            }
          }
        }
      }
    }
    frame #2 {
      # "FINALISATION"
      n605 = Quit LabVIEW(quit? (T)=TRUE ("quitter ? (V)")) -> ()
    }
  }
  n606 = property on="IMAGES FOLDER PATH" class="Path"("DisabledEnum"=T3."Disabled and Grayed Out" ("Désactivé")) -> ()  [unwired: 2 in, 2 out]
